vi "main.vi"() -> ()   [LabVIEW 2012]
uses:
  <vilib>/addons/_office/_wordsub.llb/font.ctl
  <vilib>/Utility/miscctls.llb/LVRowAndColumnTypeDef.ctl
  <vilib>/Instr/_visa.llb/VISA Configure Serial Port (Instr).vi
  <vilib>/vision/NI_Vision_Development_Module.lvlib
panel:
  in  "Algorithm":enum32{"Block Matching Algorithm"}(tab)
  in  "Correspondence Options BM":T1={"Method"=0, "Window Size"=25.0, "Minimum Disparity"=0.0, "Number of Disparity"=192.0, "Left - Right Check"=5.0, "Subpixel"=TRUE, "Invalid Disparity Replace Value"=-16.0} caption="Correspondence Options" {"Method" items=["SAD"]; "Number of Disparity" min=16.0 step=16.0; "Window Size" min=5.0 max=255.0 step=2.0}
  in  "Postfilter Options BM":T2={"Texture Threshold"=0.0, "Uniqueness Ratio"=0.0, "Speckle Window Size"=5.0, "Speckle Range"=200.0} caption="Postfilter Options" {"Speckle Range" min=0.0; "Speckle Window Size" min=0.0; "Uniqueness Ratio" min=0.0 max=100.0; "Texture Threshold" min=0.0}
  in  "Prefilter Options":T3={"Filter Type"=2, "Filter Size"=11.0, "Filter Cap"=31.0} {"Filter Type" items=["None", "Normal Response", "Sobel"]; "Filter Cap" min=1.0 max=63.0; "Filter Size" min=5.0 max=255.0 step=2.0}
  in  "Display":enum16{"Disparity Image", "Depth Image"}(ring)=enum."Depth Image"
  in  "示例图片":i32(slide) min=0 max=4 step=1 scale=0.0..4.0
  in  "开关":bool
  in  "Exit":bool
  in  "Interpolate Disparity":bool=TRUE
  in  "Depth Control":cluster{"Min Depth":dbl, "Max Depth":dbl}={"Min Depth"=0.0, "Max Depth"=40.0} {"Max Depth" min=-1.0; "Min Depth" min=-1.0}
  in  "报表信息":cluster{"font":T4, "字符串":string}={"font"={"font name"="", "font size"=12.0, "bold"=2, "italic"=2, "underline"=2, "strike through"=2, "font color"=16777222}, "字符串"=""} {"font"."font size" format="%0.2f"; "font"."strike through" items=["Strk Unchanged", "Strk Yes", "Strk No"]; "font"."underline" items=["Und Unchanged", "Und Yes", "Und No"]; "font"."italic" items=["Ital Unchanged", "Ital Yes", "Ital No"]; "font"."bold" items=["Bold Unchanged", "Bold Yes", "Bold No"]}
  in  "表格":T5={"auto format"=11, "font"={"font name"="", "font size"=0.0, "bold"=0, "italic"=0, "underline"=0, "strike through"=0, "font color"=0}, "表格 2"=[["", "", "", "", "", ""], ["2", "2.5", "7.6", "6.5", "", ""], ["", "", "", "", "", ""], ["", "", "", "", "", ""], ["", "", "", "", "", ""], ["", "", "", "", "", ""]]} {"auto format" items=["xlRangeAutoFormat3DEffects1"=13, "xlRangeAutoFormat3DEffects2"=14, "xlRangeAutoFormatAccounting1"=4, "xlRangeAutoFormatAccounting2"=5, "xlRangeAutoFormatAccounting3"=6, "xlRangeAutoFormatAccounting4"=17, "xlRangeAutoFormatClassic1"=1, "xlRangeAutoFormatClassic2"=2, "xlRangeAutoFormatClassic3"=3, "xlRangeAutoFormatColor1"=7, "xlRangeAutoFormatColor2"=8, "xlRangeAutoFormatColor3"=9, "xlRangeAutoFormatList1"=10, "xlRangeAutoFormatList2"=11, "xlRangeAutoFormatList3"=12, "xlRangeAutoFormatLocalFormat1"=15, "xlRangeAutoFormatLocalFormat2"=16, "xlRangeAutoFormatLocalFormat3"=19, "xlRangeAutoFormatLocalFormat4"=20, "xlRangeAutoFormatReport1"=21, "xlRangeAutoFormatReport2"=22, "xlRangeAutoFormatReport3"=23, "xlRangeAutoFormatReport4"=24, "xlRangeAutoFormatReport5"=25, "xlRangeAutoFormatReport6"=26, "xlRangeAutoFormatReport7"=27, "xlRangeAutoFormatReport8"=28, "xlRangeAutoFormatReport9"=29, "xlRangeAutoFormatReport10"=30, "xlRangeAutoFormatClassicPivotTable"=31, "xlRangeAutoFormatTable1"=32, "xlRangeAutoFormatTable2"=33, "xlRangeAutoFormatTable3"=34, "xlRangeAutoFormatTable4"=35, "xlRangeAutoFormatTable5"=36, "xlRangeAutoFormatTable6"=37, "xlRangeAutoFormatTable7"=38, "xlRangeAutoFormatTable8"=39, "xlRangeAutoFormatTable9"=40, "xlRangeAutoFormatTable10"=41, "xlRangeAutoFormatPTNone"=42, "xlRangeAutoFormatNone"=-4142, "xlRangeAutoFormatSimple"=-4154]; "font"."font size" format="%0.2f"; "font"."strike through" items=["Strk Unchanged", "Strk Yes", "Strk No"]; "font"."underline" items=["Und Unchanged", "Und Yes", "Und No"]; "font"."italic" items=["Ital Unchanged", "Ital Yes", "Ital No"]; "font"."bold" items=["Bold Unchanged", "Bold Yes", "Bold No"]}
  in  "内部数据显示栏值":string[][](array[string])
  out "内部数据数组":string[](array[string])
  out "Y轴（时间）":dbl
  in  "数组":dbl[][](array[numeric])=[[0.0], [0.0], [0.0], [0.0]]
  out "环境数据数组":string[](array[string])
  in  "环境数据显示栏值":string[][](array[string])
  out "Calibrating":bool=TRUE
  in  "Clean":bool
  out "报警计数":dbl
  out "果实报警数组":string[](array[string])
  out "问题叶片报警数组":string[](array[string])
  in  "颜色簇":T6={"报警没确认"=15663104, "背景色"=16448250, "消除没确认"=16777224, "报警已确认"=15331072}
  in  "消除未确认行号数组":dbl[](array[numeric])
  in  "报警已确认行号数组":dbl[](array[numeric])
  in  "报警没确认行号数组":dbl[](array[numeric])
  in  "数据显示栏值":string[][](array[string])
  in  "stop":bool
  in  "主选项卡":enum32{"主控制面板", "记录", "设置"}(tab)
  in  "子选项卡":enum32{"主监视界面", "环境数据监视界面", "内部数据监视界面", "地图"}(tab)
  in  "行驶控制":T7 {"距离" scale=0.0..50.0; "方向" scale=0.36..360.0}
  in  "测试图片":i8(slide) scale=0.0..5.0
  in  "主摄像头开关":bool
  out "花蕾":bool
  out "花朵":bool
  out "问题叶片":bool
  out "正常叶片":bool
  out "未成熟果实":bool
  out "果实":bool
  out "花蕾":dbl
  out "花朵":dbl
  out "问题叶片":dbl
  out "正常叶片":dbl
  out "未成熟果实":dbl
  out "果实":dbl
  out "主摄像头":T8(plugin-control)
  out "通信状态":T9
  out "GPS":T10={"状态"="无效GPS", "经度"="117.124598", "纬度"="34.176800", "UTC"="08时02分46秒"}
  in  "运行状态":T11={"开始时间"="00:00", "停止时间"="00:00", "小车状态"=FALSE}
  out "环境数据":T12
  out "内部数据":cluster{"电量":T13} {"电量" scale=0.0..100.0}
  in  "当前报警":i32(listbox)
  out "环境数据":dbl[][](graph)
  in  "环境数据":i32(listbox)
  in  "内部数据":i32(listbox)
  in  "WebBrowser":refnum<k7>(container) caption="地图显示窗口"
  in  "报警显示选项卡":enum32{"报警", "数据"}(tab)
  in  "当前报警列表框":i32(listbox)
  out "Rar":bool
  out "Pics":bool
  out "Execel":bool
  out "Html":bool
  in  "上传至服务器":bool
  in  "写入数据库":bool
  in  "生成报表":bool
  in  "设置选项卡":T14(tab)
  out "报警设置":i32(listbox)
  out "actual data":string
  in  "GPS状态":string[](array[string])=["初始化", "单点定位", "差分定位", "无效GPS", "固定解", "浮点解", "正在估算"]
  out "状态":string
  out "UTC时间":string
  out "GPGGA":string
  out "经度":string
  out "纬度":string
  in  "VISA resource name":refnum<visa-resource-name>="COM5"
  in  "baud rate (9600)":u32=9600
  in  "确定按钮":bool
  in  "从机数据地址":string="00"
  out "Modbus报文":string
  out "值":dbl
  in  "VISA resource name for Modbus":refnum<visa-resource-name>="COM5"
  out "发生报警":bool
  in  "报警上限":dbl(slide)=81.63265306122449 scale=0.0..100.0
  out "温度计":dbl(slide)=52.47484062973238 scale=0.0..80.0
  in  "stop 2":bool
  in  "清除报警":bool
  out "报警历史":string[][](table)
  out "报警数":i32
  out "湿度计":dbl(slide)=52.47484062973238 scale=0.0..100.0
  out "气压计":dbl(slide)=52.47484062973238 scale=0.0..120.0
  out "光度计":dbl(slide)=52.47484062973238 scale=0.0..200.0
  out "时间标识":timestamp
  out "时间字符串":string
  out "日期字符串":string
  out "Right Image":T8(plugin-control)
  out "Left Image":T8(plugin-control)
  out "Image":sgl[][](graph) caption="Depth Image"
  out "Depth":dbl caption="inches"
  # "LX"
  # "kPa"
  # "%"
  # "°C"
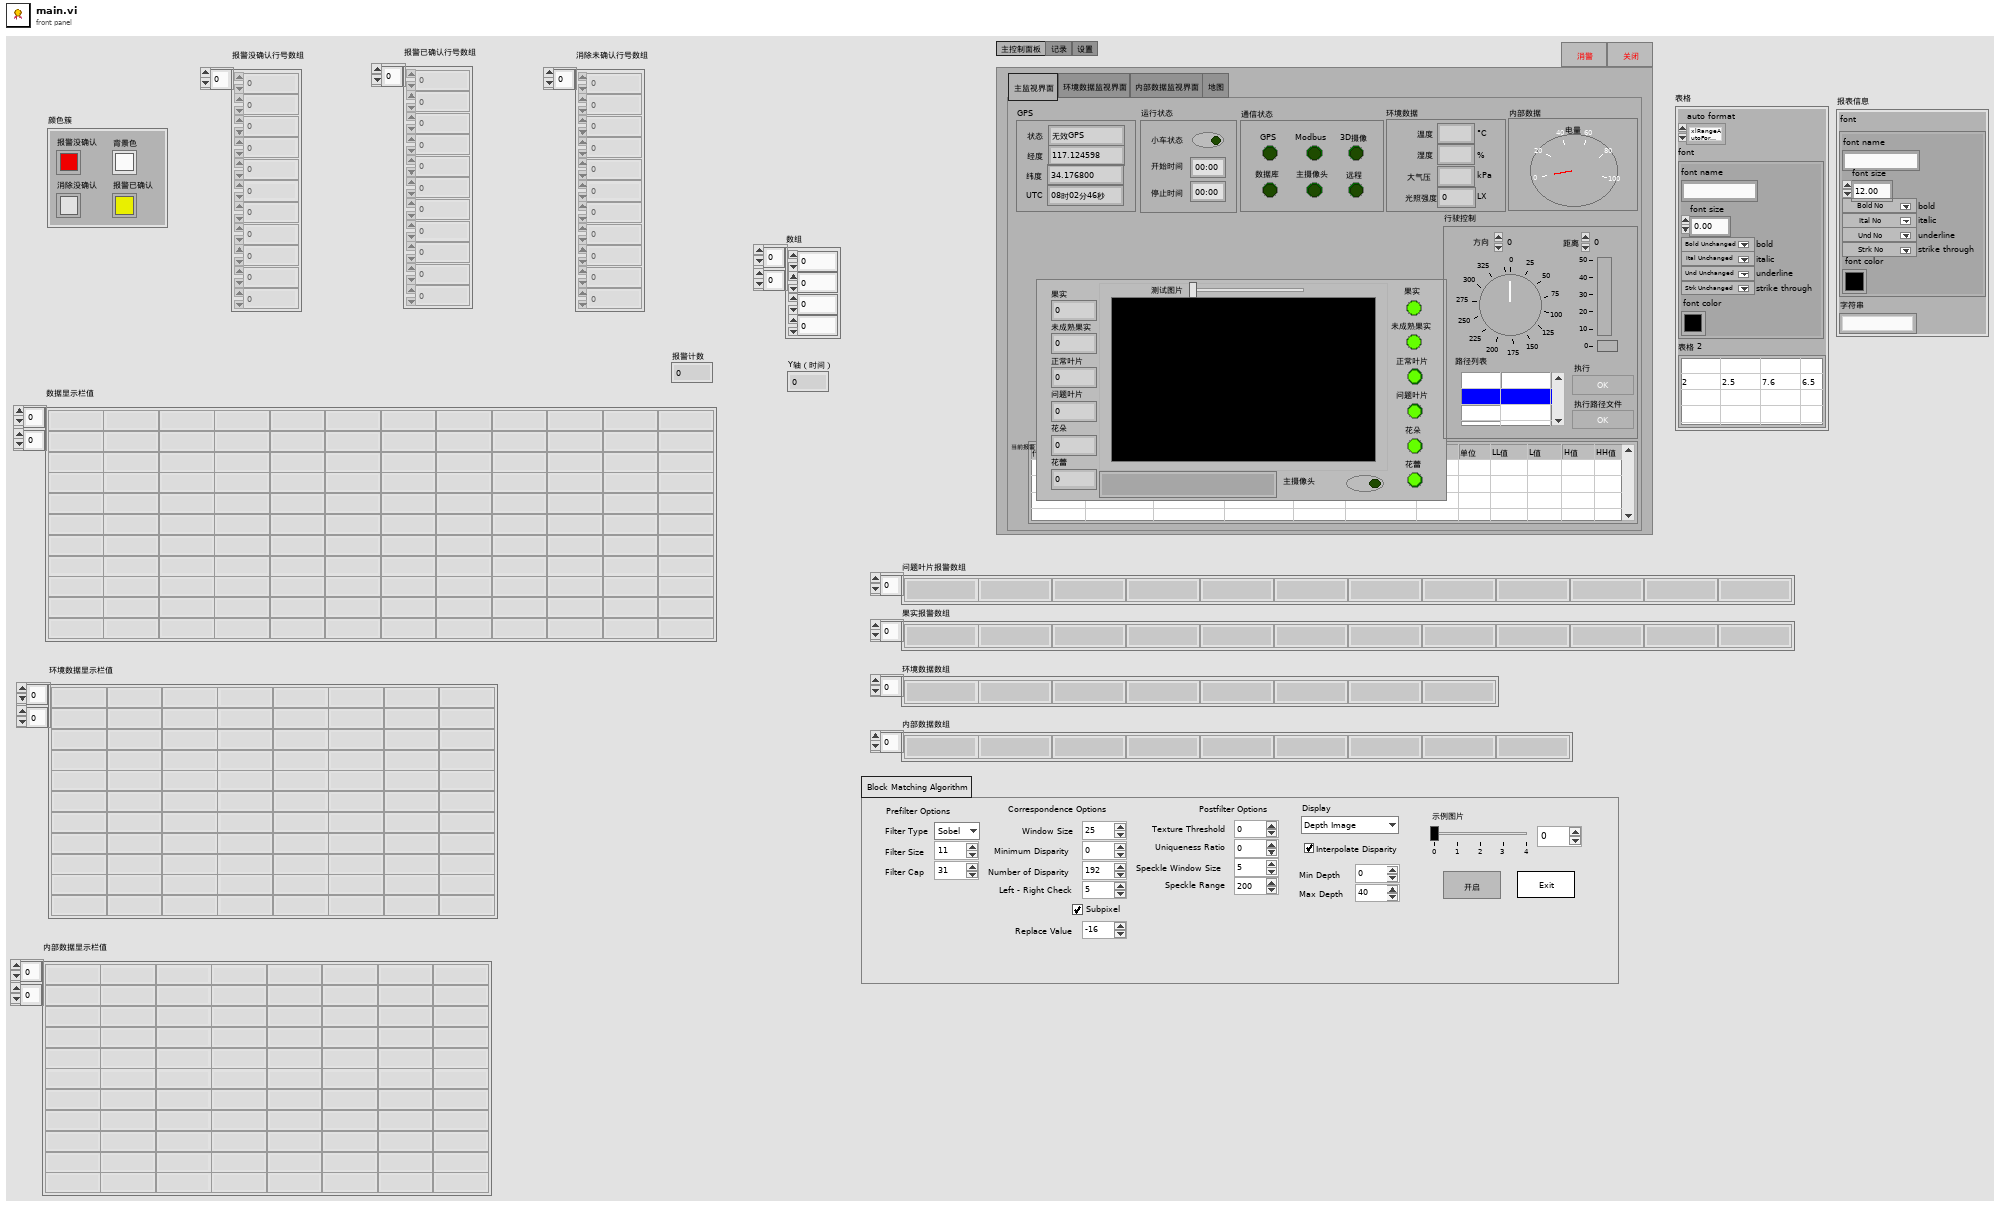
[diagram p1: front panel]
types:
  T1 = cluster{"Method":u16, "Window Size":dbl, "Minimum Disparity":dbl, "Number of Disparity":dbl, "Left - Right Check":dbl, "Subpixel":bool, "Invalid Disparity Replace Value":dbl}
  T2 = cluster{"Texture Threshold":dbl, "Uniqueness Ratio":dbl, "Speckle Window Size":dbl, "Speckle Range":dbl}
  T3 = cluster{"Filter Type":u16, "Filter Size":dbl, "Filter Cap":dbl}
  T4 = typedef "font.ctl" = cluster{"font name":string, "font size":dbl, "bold":u16, "italic":u16, "underline":u16, "strike through":u16, "font color":u32}
  T5 = cluster{"auto format":i32, "font":T4, "表格 2":string[][]}
  T6 = cluster{"报警没确认":u32, "背景色":u32, "消除没确认":u32, "报警已确认":u32}
  T7 = cluster{"方向":i32, "距离":i32, "路径列表":i32, "执行":bool, "执行路径文件":bool}
  T8 = typedef "IMAQ Image.ctl" = refnum<image>
  T9 = cluster{"GPS":bool, "数据库":bool, "Modbus":bool, "主摄像头":bool, "3D摄像":bool, "远程":bool}
  T10 = cluster{"状态":string, "经度":string, "纬度":string, "UTC":string}
  T11 = cluster{"开始时间":string, "停止时间":string, "小车状态":bool}
  T12 = cluster{"温度":dbl, "湿度":dbl, "大气压":dbl, "光照强度":dbl}
  T13 = typedef "电量.ctl" = dbl
  T14 = enum32{"报警值状态", "GPS状态", "Modbus状态", "时间状态", "3D摄像"}
  T15 = typedef "Calibration Reference Points.ctl" = cluster{"Pixel Coordinates":cluster{"X":dbl, "Y":dbl}[], "Real World Coordinates":cluster{"X":dbl, "Y":dbl}[], "Unit":T16, "Image Size":cluster{"X":u32, "Y":u32}}
  T16 = typedef "Image Unit" = enum32{"Undefined", "Angström", "Micrometer", "Millimeter", "Centimeter", "Meter", "Kilometer", "Microinch", "Inch", "Feet", "Nautical miles", "Standard miles", "Steps"}
  T17 = typedef "IMAQ Binocular Stereo Session.ctl" = refnum<k1>
  T18 = typedef "Image Type" = u32
  T19 = typedef "LVPoint32TypeDef.ctl" = cluster{"Horizontal":i32, "Vertical":i32}
  T20 = cluster{"Number of Disparity":dbl, "Number of Disparity":dbl}
  T21 = typedef "LVRowAndColumnTypeDef.ctl" = cluster{"Row":i32, "Column":i32}
  T22 = cluster{"状态":string, "经度":string, "纬度":string, "UTC时间":string}
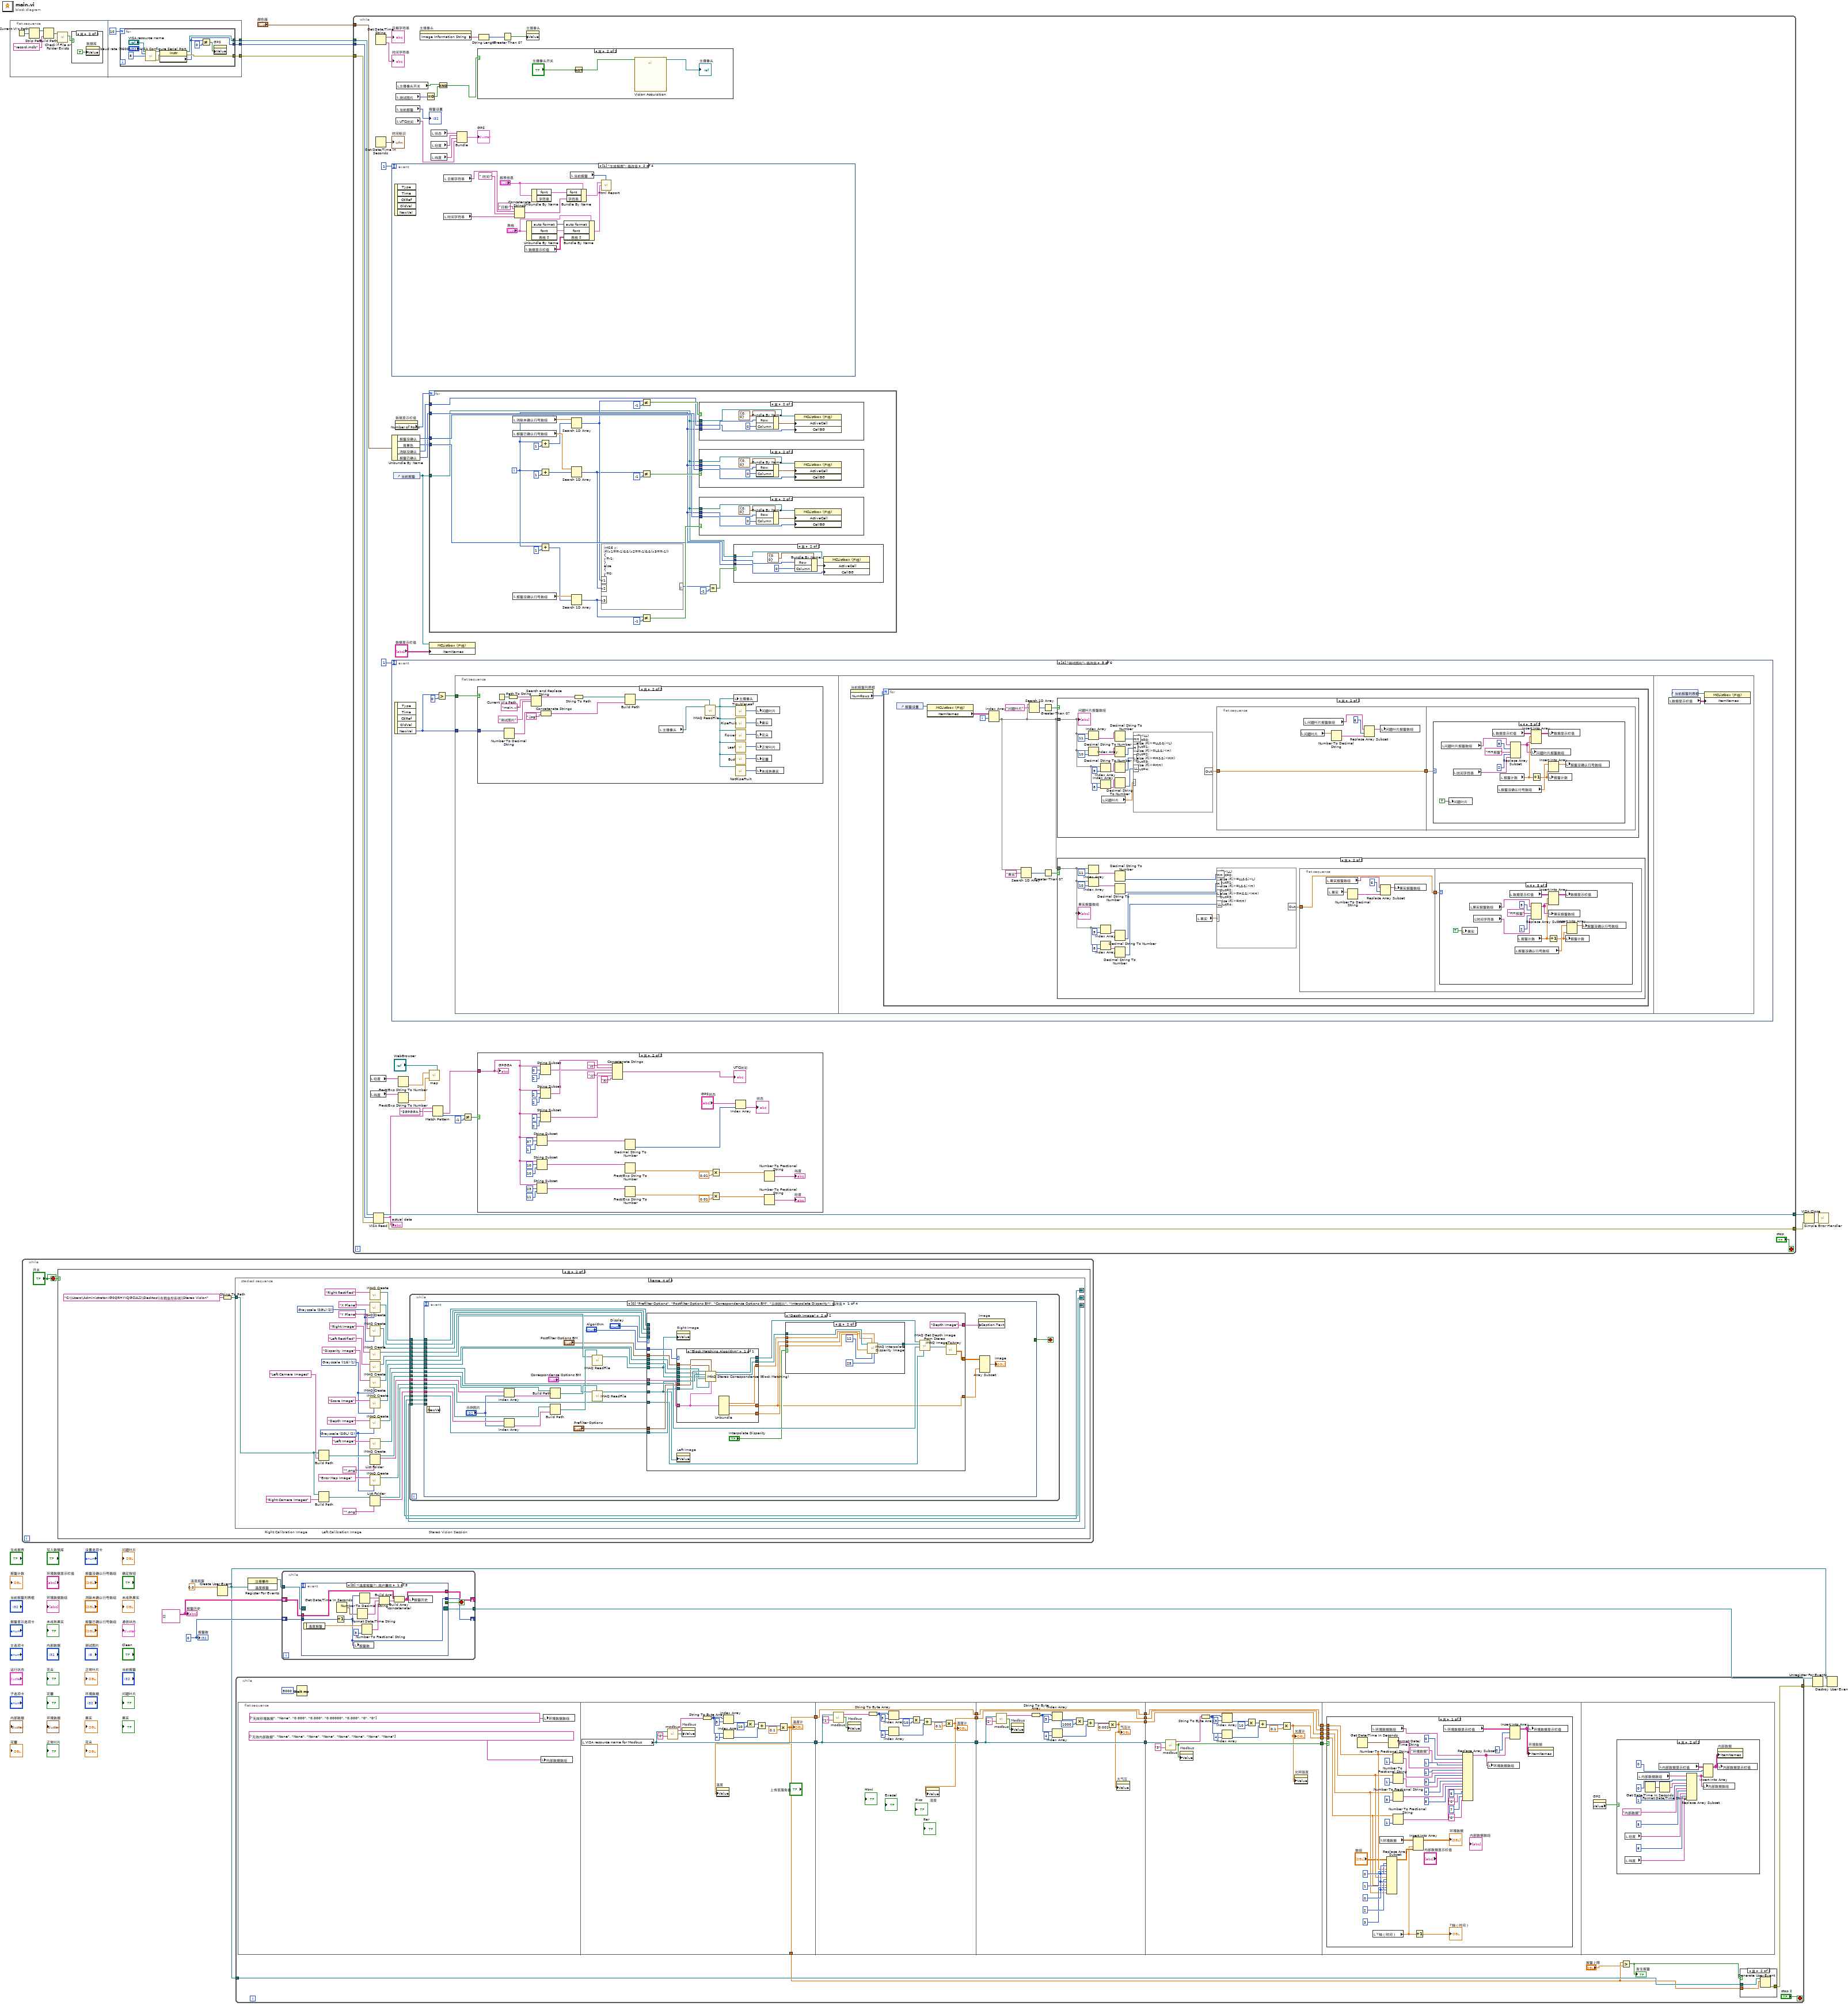
[diagram p0: block diagram]
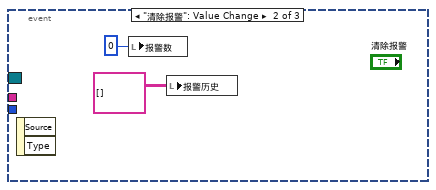
[diagram p2: hidden frame]
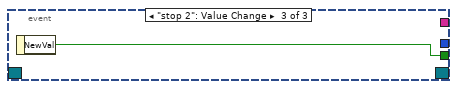
[diagram p3: hidden frame]
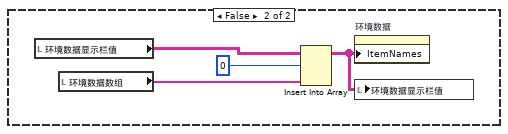
[diagram p4: hidden frame]
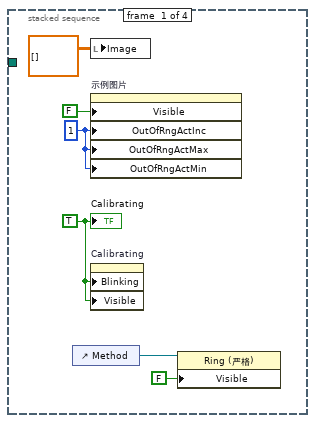
[diagram p8: hidden frame]
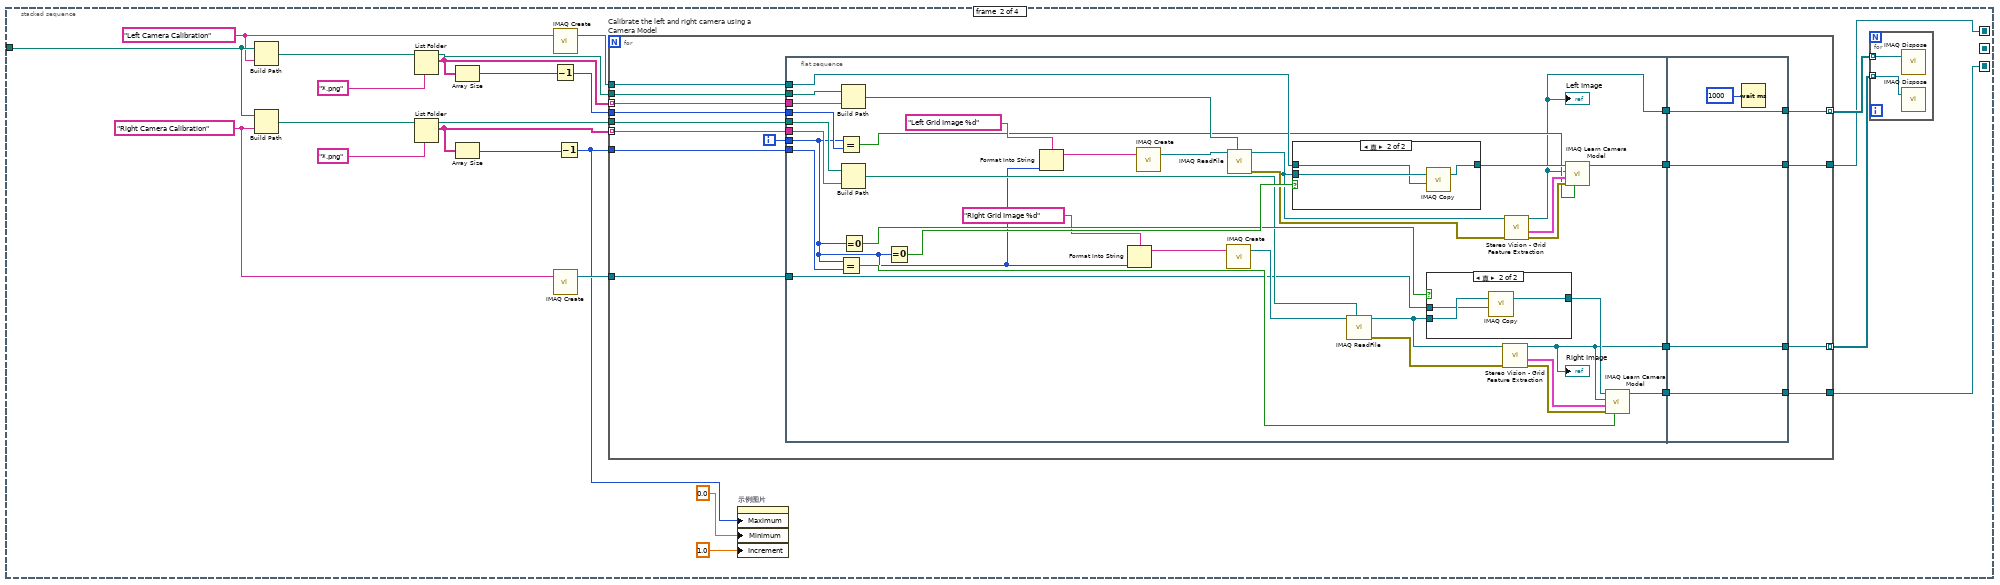
[diagram p9: hidden frame]
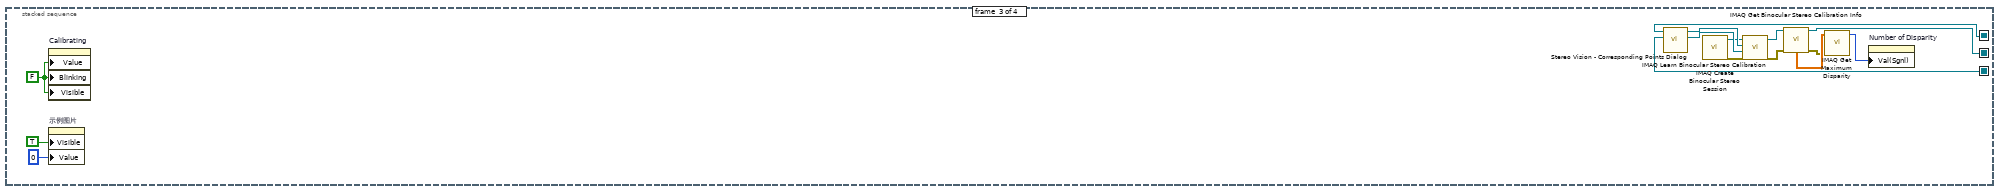
[diagram p12: hidden frame]
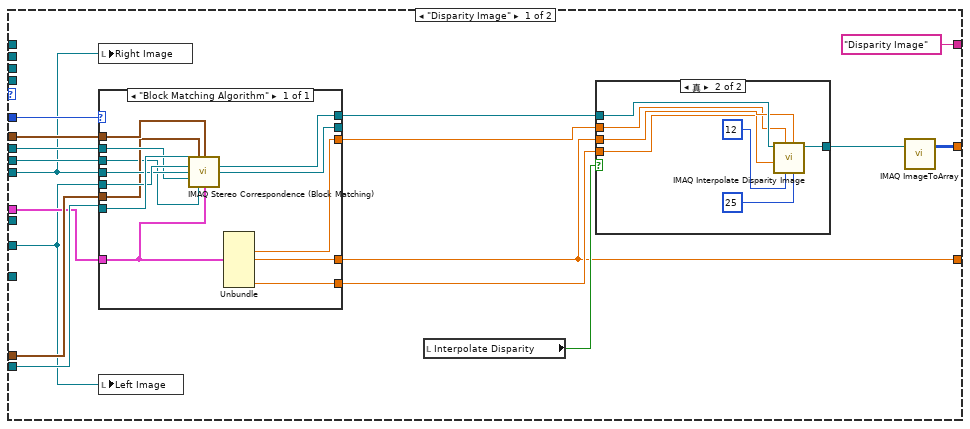
[diagram p13: hidden frame]
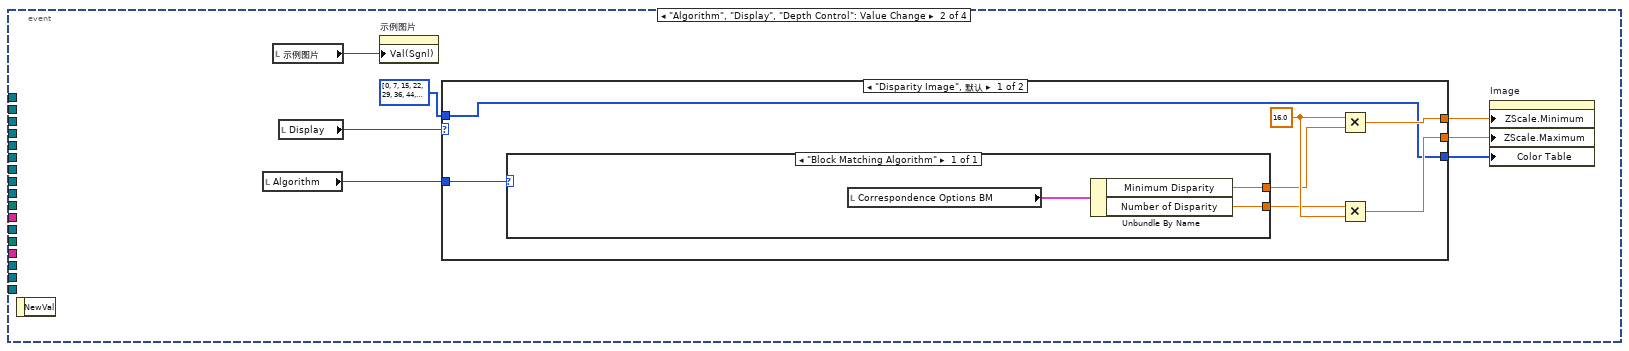
[diagram p16: hidden frame]
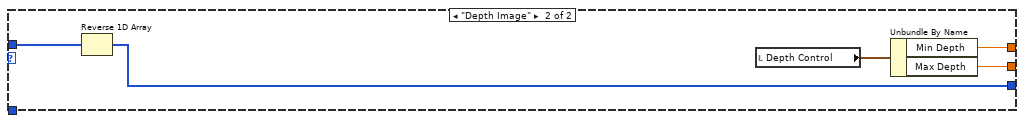
[diagram p17: hidden frame]
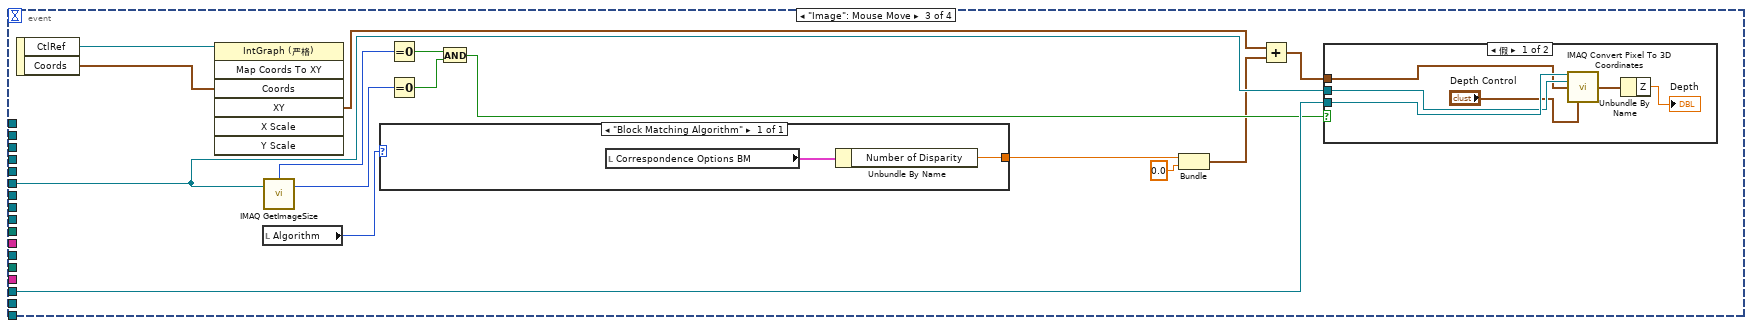
[diagram p18: hidden frame]
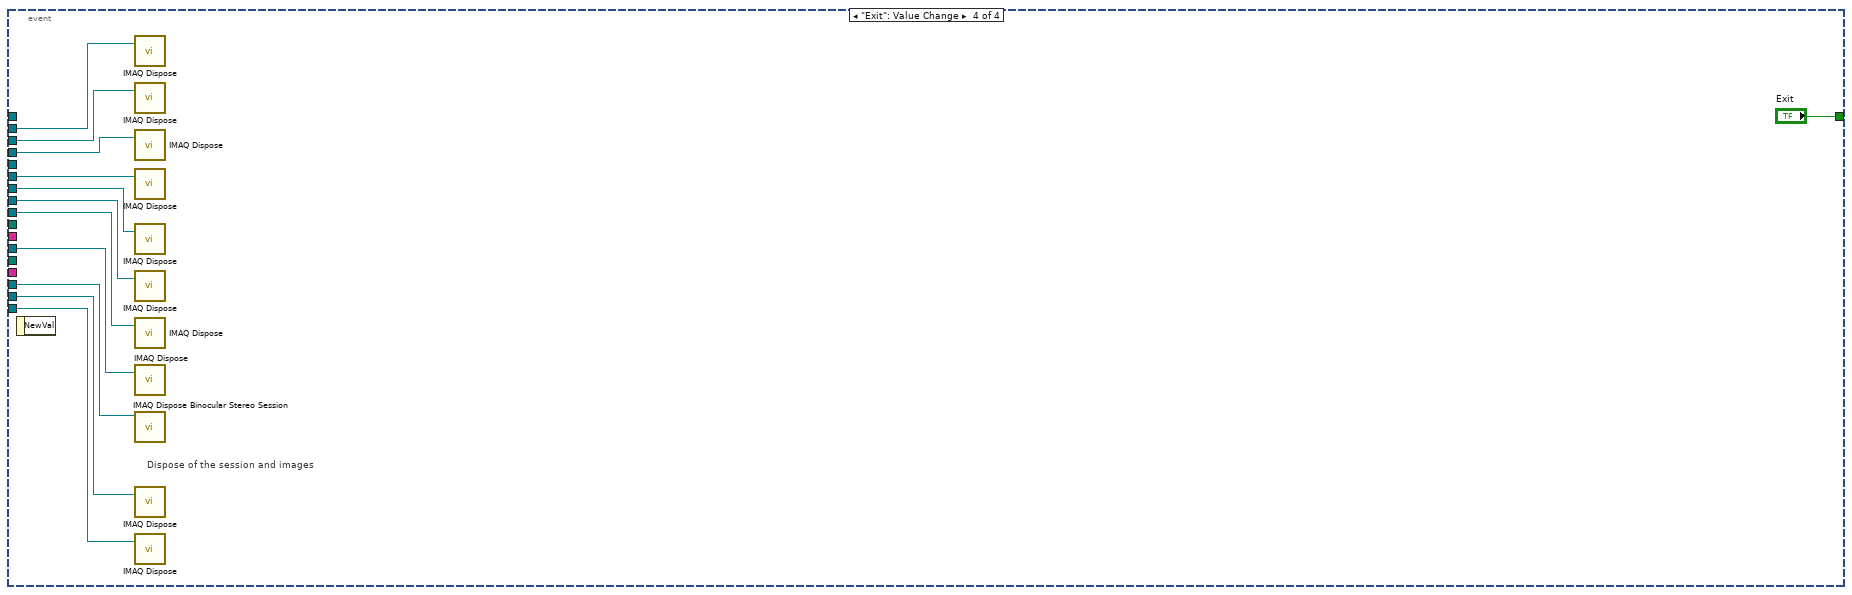
[diagram p20: hidden frame]
diagram:
  w6 = string[][] [] ("报警历史")
  w8 = 0.0  # 温度报警
  w4 = 0
  n1 = flat-sequence {
    tunnel: [w26] -> w12
    tunnel: [w25] -> w11
    tunnel: [w24] -> w10
    frame #0 {
      n2 = Current VI's Path() -> (path=w18:path)
      n3 = Strip Path(path=w18) -> (stripped path=w19:path)  [unwired: 1 out]
      n4 = Build Path(base path=w19, name or relative path="record.mdb") -> (appended path=w20:path)
      n5 = call <vilib>:"Check if File or Folder Exists.vi"("path"=w20) -> ("file or folder exists?"=w16:bool)  [unwired: 8 in, 2 out]
      n6 = case shown="真" w16 {
        frame False {
          n7 = property on="数据库" class="Bool (严格)"("Value"=FALSE) -> ()  [unwired: 2 in, 2 out]
        }
        frame True {
          n8 = property on="数据库" class="Bool (严格)"("Value"=TRUE) -> ()  [unwired: 2 in, 2 out]
        }
      }
    }
    frame #1 {
      n9 = for {
        N: 10 ("offset (0)") -> [_]
        tunnel: [w32] -> w26
        tunnel: [w30] -> w24
        tunnel: [w31] -> w25
        n10 = call-poly "VISA Configure Serial Port"("VISA resource name"="VISA resource name", "baud rate (9600)"="baud rate (9600)", "data bits (8)"=u16 8) -> ("VISA resource name out"=w28:refnum<visa-resource-name>, "error out"=w36:errorcluster)  [unwired: 3 in, 8 out]
        n11 = property class="Instr"(reference=w28, error in=w36) -> (reference out=w32:refnum<visa-resource-name>, error out=w31:errorcluster, "Serial Settings:Number of Bytes at Serial Port"=w30:u32)
        n12 = Not Equal?(x=w30, y=u32 0) -> (x != y?=w27:bool)
        n13 = property on="GPS" class="Bool (严格)"("Value"=w27) -> ()  [unwired: 2 in, 2 out]
      }
    }
  }
  n14 = while {
    stop <- "开关" stop-if-true
    n15 = case shown="真" "开关" {
      frame False {
      }
      frame True {
        # "Stereo Vision Session"
        # "Right Calibration Image"
        # "Left Calibration Image"
        n16 = String To Path(string="C:\\Users\\Administrator.IG0QRHYICJGCULZ\\Desktop\\车载监控系统\\Stereo Vision" ("name or relative path")) -> (path=w38:path)
        n17 = stacked-sequence {
          seq-local: [_ w53 _ _] -> [_ _ w139 w155]
          seq-local: [_ w52 _ _] -> [_ _ w138 w154]
          seq-local: [_ _ w137 _] -> [_ _ _ w153]
          tunnel: w38 -> [_ w65 _ w187]
          frame #0 {
            w43 = u8 1 ("Response to Value Outside Limits:Maximum")
            w44 = TRUE ("Calibrating")
            n18 = control-ref of="Method"() -> (w42:refnum<vi>)
            n19 = local write "Image"(sgl[][] [] ("Image")) -> ()
            n20 = property on="示例图片" class="Slide (严格)"("Visible"=FALSE, "OutOfRngActInc"=w43, "OutOfRngActMax"=w43, "OutOfRngActMin"=w43) -> ()  [unwired: 2 in, 2 out]
            n21 = property on="Calibrating" class="Bool (严格)"("Blinking"=w44, "Visible"=w44) -> ()  [unwired: 2 in, 2 out]
            n22 = property class="Ring (严格)"(reference=w42, "Visible"=FALSE) -> ()  [unwired: 1 in, 2 out]
            "Calibrating" <- w44
          }
          frame #1 {
            w63 = "Right Camera Calibration" ("name or relative path")
            w64 = "Left Camera Calibration" ("name or relative path")
            n23 = Build Path(base path=w65, name or relative path=w64) -> (appended path=w68:path)
            n24 = Build Path(base path=w65, name or relative path=w63) -> (appended path=w66:path)
            n25 = List Folder(path=w68, pattern="*.png") -> (path out=w62:path, filenames=w59:string[])  [unwired: 1 in, 3 out]
            n26 = List Folder(path=w66, pattern="*.png") -> (path out=w61:path, filenames=w56:string[])  [unwired: 1 in, 3 out]
            n27 = Array Size(array=w59) -> (size(s)=w67:i32)
            n28 = Array Size(array=w56) -> (size(s)=w51:i32)
            n29 = call "IMAQ Create"("Image Name"=w64) -> ("New Image"=w60:T8)  [unwired: 3 in, 2 out]
            n30 = Decrement(x=w67) -> (x-1=w58:i32)
            n31 = call "IMAQ Create"("Image Name"=w63) -> ("New Image"=w57:T8)  [unwired: 3 in, 2 out]
            n32 = Decrement(x=w51) -> (x-1=w50:i32)
            n33 = for "Calibrate the left and right camera using a Camera Model" {
              tunnel: w59 -> [w86] mode=indexing
              tunnel: w56 -> [w81] mode=indexing
              tunnel: w62 -> [w87]
              tunnel: w61 -> [w82]
              tunnel: w60 -> [w85]
              tunnel: [w84] -> w53
              tunnel: w58 -> [w83]
              tunnel: [w80] -> w52
              tunnel: w57 -> [w79]
              tunnel: w50 -> [w78]
              tunnel: [w77] -> w54 mode=indexing
              tunnel: [w76] -> w55 mode=indexing
              i -> [w75]
              n34 = flat-sequence {
                tunnel: w87 -> [w118]
                tunnel: w86 -> [w116]
                tunnel: w85 -> [w114]
                tunnel: w83 -> [w109]
                tunnel: w82 -> [w97]
                tunnel: w81 -> [w96]
                tunnel: w79 -> [w94]
                tunnel: w78 -> [w93]
                tunnel: w75 -> [w92]
                tunnel: [w110] -> w74
                tunnel: [w95] -> w73
                tunnel: [w88] -> w72
                tunnel: [w90] -> w71
                tunnel: [w132] -> w76
                tunnel: [w133] -> w77
                tunnel: [w134] -> w80
                tunnel: [w135] -> w84
                tunnel: w74 -> [w135]
                tunnel: w73 -> [w134]
                tunnel: w72 -> [w133]
                tunnel: w71 -> [w132]
                frame #0 {
                  n35 = Equal?(x=w92, y=w109) -> (x = y?=w108:bool)
                  n36 = Equal?(x=w92, y=w93) -> (x = y?=w107:bool)
                  n37 = Build Path(base path=w118, name or relative path=w116) -> (appended path=w119:path)
                  n38 = Build Path(base path=w97, name or relative path=w96) -> (appended path=w101:path)
                  n39 = Equal To 0?(x=w92) -> (x = 0?=w104:bool)
                  n40 = Equal To 0?(x=w92) -> (x = 0?=w113:bool)
                  n41 = Format Into String(format string="Left Grid Image %d" ("name or relative path"), w92) -> (resulting string=w115:string)  [unwired: 2 in, 1 out]
                  n42 = Format Into String(format string="Right Grid Image %d" ("name or relative path"), w92) -> (resulting string=w103:string)  [unwired: 2 in, 1 out]
                  n43 = call "IMAQ Create"("Image Name"=w115) -> ("New Image"=w122:T8)  [unwired: 3 in, 2 out]
                  n44 = call "IMAQ Create"("Image Name"=w103) -> ("New Image"=w98:T8)  [unwired: 3 in, 2 out]
                  n45 = call "IMAQ ReadFile"("File Path"=w119, "Image"=w122) -> ("error out"=w111:errorcluster, "Image Out"=w91:T8)  [unwired: 3 in, 5 out]
                  n46 = case shown="真" w113 {
                    tunnel: w91 -> [_ w130]
                    tunnel: w114 -> [w127 w129]
                    tunnel: [w127 w128] -> w112
                    frame False {
                    }
                    frame True {
                      n47 = call "IMAQ Copy"("Image Dst"=w129, "Image Src"=w130) -> ("Image Dst Out"=w128:T8)  [unwired: 1 in, 4 out]
                    }
                  }
                  n48 = call "IMAQ ReadFile"("File Path"=w101, "Image"=w98) -> ("error out"=w106:errorcluster, "Image Out"=w89:T8)  [unwired: 3 in, 5 out]
                  n49 = case shown="真" w104 {
                    tunnel: w89 -> [_ w126]
                    tunnel: w94 -> [w123 w125]
                    tunnel: [w123 w124] -> w105
                    frame False {
                    }
                    frame True {
                      n50 = call "IMAQ Copy"("Image Dst"=w125, "Image Src"=w126) -> ("Image Dst Out"=w124:T8)  [unwired: 1 in, 4 out]
                    }
                  }
                  n51 = call "Stereo Vision - Grid Feature Extraction.vi"("error in (no error)"=w106, "Image in"=w89) -> ("error out"=w99:errorcluster, "Reference Points"=w100:T15, "Image (dup)"=w88:T8)  [unwired: 7 out]
                  "Right Image" <- w88
                  n52 = call "Stereo Vision - Grid Feature Extraction.vi"("error in (no error)"=w111, "Image in"=w91) -> ("error out"=w121:errorcluster, "Reference Points"=w120:T15, "Image (dup)"=w90:T8)  [unwired: 7 out]
                  "Left Image" <- w90
                  n53 = call "IMAQ Learn Camera Model"("Add Points and Learn (True)"=w108, "error in (no error)"=w121, "Reference Points"=w120, "Image"=w90, "Calibration Template Image"=w112) -> ("Calibration Template Image Out"=w110:T8)  [unwired: 1 in, 5 out]
                  n54 = call "IMAQ Learn Camera Model"("Add Points and Learn (True)"=w107, "error in (no error)"=w99, "Reference Points"=w100, "Image"=w88, "Calibration Template Image"=w105) -> ("Calibration Template Image Out"=w95:T8)  [unwired: 1 in, 5 out]
                }
                frame #1 {
                  n55 = Wait (ms)(milliseconds to wait=u32 1000 ("millisecond timer value")) -> ()  [unwired: 1 out]
                }
              }
            }
            n56 = property on="示例图片" class="Slide (严格)"("Maximum"=w50, "Minimum"=0.0 ("Data Entry Limits:Minimum"), "Increment"=1.0 ("Data Entry Limits:Increment")) -> ()  [unwired: 2 in, 2 out]
            n57 = for {
              tunnel: w55 -> [w70] mode=indexing
              tunnel: w54 -> [w69] mode=indexing
              n58 = call "IMAQ Dispose"("Image"=w70) -> ()  [unwired: 2 in, 4 out]
              n59 = call "IMAQ Dispose"("Image"=w69) -> ()  [unwired: 2 in, 4 out]
            }
          }
          frame #2 {
            w150 = FALSE ("Calibrating")
            n60 = property on="Calibrating" class="Bool (严格)"("Value"=w150, "Blinking"=w150, "Visible"=w150) -> ()  [unwired: 2 in, 2 out]
            n61 = property on="示例图片" class="Slide (严格)"("Visible"=TRUE, "Value"=0 ("Value (Signaling)")) -> ()  [unwired: 2 in, 2 out]
            n62 = call "Stereo Vision - Corresponding Points Dialog.vi"("Right Image in"=w138, "Left Image in"=w139) -> ("Right Image out"=w143:T8, "Left Image out"=w142:T8)  [unwired: 8 out]
            n63 = call "IMAQ Create Binocular Stereo Session"() -> ("error out"=w141:errorcluster, "Binocular Stereo Session Out"=w140:T17)  [unwired: 1 in, 9 out]
            n64 = call "IMAQ Learn Binocular Stereo Calibration"("error in (no error)"=w141, "Right Calibration Template"=w143, "Left Calibration Template"=w142, "Binocular Stereo Session"=w140) -> ("error out"=w147:errorcluster, "Binocular Stereo Session (dup)"=w146:T17)  [unwired: 1 in, 5 out]
            n65 = call "IMAQ Get Binocular Stereo Calibration Info"("Binocular Stereo Session"=w146, "error in (no error)"=w147) -> ("Binocular Stereo Session (dup)"=w137:T17, "Q Matrix"=w145:dbl[][], "error out"=w144:errorcluster)  [unwired: 11 out]
            n66 = call "IMAQ Get Maximum Disparity"("error in (no error)"=w144, "Q Matrix"=w145) -> ("Max. Disparity"=w136:i32)  [unwired: 2 in, 7 out]
            n67 = property on="Number of Disparity" class="DigNum (严格)"("Val(Sgnl)"=w136) -> ()  [unwired: 2 in, 2 out]
          }
          frame #3 {
            w160 = T18 2 items=["Grayscale (U8)", "Grayscale (I16)", "Grayscale (SGL)", "Complex (CSG)", "RGB (U32)", "HSL (U32)", "RGB (U64)", "Grayscale (U16)"] ("Image Type")
            w161 = T18 2 items=["Grayscale (U8)", "Grayscale (I16)", "Grayscale (SGL)", "Complex (CSG)", "RGB (U32)", "HSL (U32)", "RGB (U64)", "Grayscale (U16)"] ("Image Type")
            w162 = T18 1 items=["Grayscale (U8)", "Grayscale (I16)", "Grayscale (SGL)", "Complex (CSG)", "RGB (U32)", "HSL (U32)", "RGB (U64)", "Grayscale (U16)"] ("Image Type")
            n68 = Build Path(base path=w187, name or relative path="Left Camera Images") -> (appended path=w186:path)
            n69 = Build Path(base path=w187, name or relative path="Right Camera Images") -> (appended path=w183:path)
            n70 = call "IMAQ Create"("Image Name"="Right Rectified") -> ("New Image"=w156:T8)  [unwired: 3 in, 2 out]
            n71 = call "IMAQ Create"("Image Name"="X Plane", "Image Type"=w160) -> ("New Image"=w164:T8)  [unwired: 2 in, 2 out]
            n72 = call "IMAQ Create"("Image Name"="Y Plane", "Image Type"=w160) -> ("New Image"=w163:T8)  [unwired: 2 in, 2 out]
            n73 = call "IMAQ Create"("Image Name"="Right Image") -> ("New Image"=w175:T8)  [unwired: 3 in, 2 out]
            n74 = call "IMAQ Create"("Image Name"="Left Rectified") -> ("New Image"=w157:T8)  [unwired: 3 in, 2 out]
            n75 = call "IMAQ Create"("Image Name"="Disparity Image", "Image Type"=w162) -> ("New Image"=w173:T8)  [unwired: 2 in, 2 out]
            n76 = call "IMAQ Create"("Image Name"="Score Image", "Image Type"=w162) -> ("New Image"=w171:T8)  [unwired: 2 in, 2 out]
            n77 = call "IMAQ Create"("Image Name"="Depth Image", "Image Type"=w161) -> ("New Image"=w169:T8)  [unwired: 2 in, 2 out]
            n78 = call "IMAQ Create"("Image Name"="Left Image") -> ("New Image"=w178:T8)  [unwired: 3 in, 2 out]
            n79 = List Folder(path=w186, pattern="*.png") -> (path out=w180:path, filenames=w182:string[])  [unwired: 1 in, 3 out]
            n80 = call "IMAQ Create"("Image Name"="Error Map Image", "Image Type"=w161) -> ("New Image"=w167:T8)  [unwired: 2 in, 2 out]
            n81 = List Folder(path=w183, pattern="*.png") -> (path out=w179:path, filenames=w181:string[])  [unwired: 1 in, 3 out]
            n82 = while {
              tunnel: w182 -> [w205]
              tunnel: w181 -> [w204]
              tunnel: w180 -> [w203]
              tunnel: w179 -> [w202]
              tunnel: w178 -> [w201]
              tunnel: w153 -> [w200]
              tunnel: w175 -> [w199]
              tunnel: w173 -> [w198]
              tunnel: w171 -> [w197]
              tunnel: w169 -> [w196]
              tunnel: w167 -> [w195]
              tunnel: w164 -> [w194]
              tunnel: w163 -> [w193]
              tunnel: w155 -> [w191]
              tunnel: w154 -> [w190]
              tunnel: w157 -> [w189]
              tunnel: w156 -> [w188]
              stop <- w192 stop-if-true
              n83 = event shown="[0] \"Prefilter Options\", \"Postfilter Options BM\", \"Correspondence Options BM\", \"示例图片\", \"Interpolate Disparity\": 值改变" {
                selector: _ -> [_ _ _ _]
                dyn-events: _ -> [_ _ _ _]
                timeout: _ -> [_ _ _ _]
                tunnel: w205 -> [w232 _ _ _]
                tunnel: w204 -> [w230 _ _ _]
                tunnel: w203 -> [w233 _ _ _]
                tunnel: w202 -> [w231 _ _ _]
                tunnel: w201 -> [w228 _ _ w372]
                tunnel: w200 -> [w225 _ w353 w364]
                tunnel: w199 -> [w223 _ _ w371]
                tunnel: w198 -> [w222 _ w352 w370]
                tunnel: w197 -> [w218 _ _ w369]
                tunnel: w196 -> [w217 _ _ w368]
                tunnel: w195 -> [w215 _ _ w367]
                tunnel: w194 -> [w214 _ _ w366]
                tunnel: w193 -> [w213 _ _ w365]
                tunnel: [_ _ _ "Exit"] -> w192
                tunnel: w191 -> [_ _ _ w363]
                tunnel: w190 -> [_ _ _ w362]
                tunnel: w189 -> [w212 _ _ _]
                tunnel: w188 -> [w211 _ _ _]
                event "Prefilter Options", "Postfilter Options BM", "Correspondence Options BM", "示例图片", "Interpolate Disparity": Value Change {
                  n84 = event-data() -> ()  [unwired: 2 out]
                  n85 = Index Array(array=w232, index="示例图片") -> (element=w236:string)
                  n86 = Index Array(array=w230, index="示例图片") -> (element=w235:string)
                  n87 = Build Path(base path=w233, name or relative path=w236) -> (appended path=w234:path)
                  n88 = Build Path(base path=w231, name or relative path=w235) -> (appended path=w224:path)
                  n89 = call "IMAQ ReadFile"("File Path"=w224, "Image"=w223) -> ("Image Out"=w209:T8)  [unwired: 3 in, 6 out]
                  n90 = call "IMAQ ReadFile"("File Path"=w234, "Image"=w228) -> ("Image Out"=w210:T8)  [unwired: 3 in, 6 out]
                  n91 = case shown="\"Depth Image\"" "Display" {
                    tunnel: w225 -> [w251 w290]
                    tunnel: w210 -> [w239 w284]
                    tunnel: w209 -> [w238 w283]
                    tunnel: w222 -> [w250 w289]
                    tunnel: "Algorithm" -> [w247 w293]
                    tunnel: "Postfilter Options BM" -> [w253 w292]
                    tunnel: "Prefilter Options" -> [w252 w291]
                    tunnel: "Correspondence Options BM" -> [w249 w287]
                    tunnel: [w240 w276] -> w208
                    tunnel: ["Disparity Image" ("Caption.Text") "Depth Image" ("Caption.Text")] -> w216
                    tunnel: w218 -> [w246 w288]
                    tunnel: w217 -> [_ w294]
                    tunnel: w215 -> [_ w285]
                    tunnel: w214 -> [_ _]
                    tunnel: w213 -> [_ _]
                    tunnel: w212 -> [_ _]
                    tunnel: w211 -> [_ _]
                    tunnel: [w237 w275] -> w206
                    frame "Disparity Image" {
                      n92 = local write "Right Image"(w238) -> ()
                      n93 = case shown="\"Block Matching Algorithm\"" w247 {
                        tunnel: w251 -> [w274]
                        tunnel: w239 -> [w273]
                        tunnel: w238 -> [w272]
                        tunnel: w250 -> [w271]
                        tunnel: [w270] -> w245
                        tunnel: w253 -> [w269]
                        tunnel: w252 -> [w268]
                        tunnel: w249 -> [w265]
                        tunnel: w246 -> [w267]
                        tunnel: [w266] -> _
                        tunnel: [w262] -> w244
                        tunnel: [w264] -> w243
                        tunnel: [w263] -> w237
                        frame "Block Matching Algorithm" {
                          n94 = call "IMAQ Stereo Correspondence (Block Matching)"("Binocular Stereo Session"=w274, "Prefilter Options"=w268, "Postfilter Options"=w269, "Left Image In"=w273, "Right Image In"=w272, "Disparity Image In"=w271, "Score Image In"=w267, "Correspondence Options"=w265) -> ("Disparity Image Out"=w270:T8, "Score Image Out"=w266:T8)  [unwired: 1 in, 5 out]
                          n95 = Unbundle(w265) -> ("Minimum Disparity"=w264:dbl, "Number of Disparity"=w263:dbl, "Invalid Disparity Replace Value"=w262:dbl)  [unwired: 4 out]
                        }
                      }
                      n96 = local write "Left Image"(w239) -> ()
                      n97 = local read "Interpolate Disparity"() -> (w242:bool)
                      n98 = case shown="真" w242 {
                        tunnel: w245 -> [w254 w261]
                        tunnel: [w254 w260] -> w241
                        tunnel: w237 -> [_ w259]
                        tunnel: w243 -> [_ w258]
                        tunnel: w244 -> [_ w257]
                        frame False {
                        }
                        frame True {
                          n99 = call "IMAQ Interpolate Disparity Image"("Sampling Frequency"=25, "Number of Disparities"=w259, "Order"=12, "Minimum Disparity"=w258, "Invalid Disparity Value"=w257, "Image Src"=w261) -> ("Image Dst Out"=w260:T8)  [unwired: 2 in, 3 out]
                        }
                      }
                      n100 = call "IMAQ ImageToArray"("Image"=w241) -> ("Image Pixels (I16)"=w240:i16[][])  [unwired: 2 in, 5 out]
                    }
                    frame "Depth Image" {
                      n101 = property on="Right Image" class="ImageControl"("Value"=w283) -> ()  [unwired: 2 in, 2 out]
                      n102 = case shown="\"Block Matching Algorithm\"" w293 {
                        tunnel: w290 -> [w316]
                        tunnel: w284 -> [w315]
                        tunnel: w283 -> [w314]
                        tunnel: w289 -> [w313]
                        tunnel: [w312] -> w281
                        tunnel: w292 -> [w311]
                        tunnel: w291 -> [w310]
                        tunnel: w288 -> [w309]
                        tunnel: w287 -> [w307]
                        tunnel: [w308] -> w286
                        tunnel: [w306] -> w280
                        tunnel: [w305] -> w279
                        tunnel: [w304] -> w275
                        frame "Block Matching Algorithm" {
                          n103 = call "IMAQ Stereo Correspondence (Block Matching)"("Binocular Stereo Session"=w316, "Prefilter Options"=w310, "Postfilter Options"=w311, "Left Image In"=w315, "Right Image In"=w314, "Disparity Image In"=w313, "Score Image In"=w309, "Correspondence Options"=w307) -> ("Binocular Stereo Session (dup)"=w308:T17, "Disparity Image Out"=w312:T8)  [unwired: 1 in, 5 out]
                          n104 = Unbundle(w307) -> ("Minimum Disparity"=w305:dbl, "Number of Disparity"=w304:dbl, "Invalid Disparity Replace Value"=w306:dbl)  [unwired: 4 out]
                        }
                      }
                      n105 = property on="Left Image" class="ImageControl"("Value"=w284) -> ()  [unwired: 2 in, 2 out]
                      n106 = case shown="真" "Interpolate Disparity" {
                        tunnel: [w296 w303] -> w282
                        tunnel: w281 -> [w296 w302]
                        tunnel: w280 -> [_ w301]
                        tunnel: w279 -> [_ w300]
                        tunnel: w275 -> [_ w299]
                        frame False {
                        }
                        frame True {
                          n107 = call "IMAQ Interpolate Disparity Image"("Sampling Frequency"=25, "Number of Disparities"=w299, "Order"=12, "Minimum Disparity"=w300, "Invalid Disparity Value"=w301, "Image Src"=w302) -> ("Image Dst Out"=w303:T8)  [unwired: 2 in, 3 out]
                        }
                      }
                      n108 = call "IMAQ Get Depth Image From Stereo"("Error Map In"=w285, "Depth Image In"=w294, "Disparity Image"=w282, "Binocular Stereo Session"=w286) -> ("Depth Image Out"=w277:T8)  [unwired: 3 in, 4 out]
                      n109 = call "IMAQ ImageToArray"("Image"=w277) -> ("Image Pixels (Float)"=w276:sgl[][])  [unwired: 2 in, 5 out]
                    }
                  }
                  n110 = property on="Image" class="IntGraph (严格)"("Caption.Text"=w216) -> ()  [unwired: 2 in, 2 out]
                  n111 = Array Subset(array=w208, index (col)=w206) -> (→"Image":sgl[][])  [unwired: 3 in]
                }
                event "Correspondence Options BM.Minimum Disparity", "Correspondence Options BM.Number of Disparity", "Algorithm", "Display", "Depth Control": Value Change {
                  n112 = event-data() -> ()  [unwired: 2 out]
                  n113 = local read "Algorithm"() -> (w323:enum32{"Block Matching Algorithm"})
                  n114 = local read "示例图片"() -> (w317:i32)
                  n115 = local read "Display"() -> (w320:enum16{"Disparity Image", "Depth Image"})
                  n116 = property on="示例图片" class="Slide (严格)"("Val(Sgnl)"=w317) -> ()  [unwired: 2 in, 2 out]
                  n117 = case shown="\"Disparity Image\", 默认" w320 {
                    tunnel: w323 -> [w330 _]
                    tunnel: [w326 w335] -> w322
                    tunnel: [w325 w334] -> w321
                    tunnel: u32[] [0, 7, 15, 22, 29, 36, 44, 51, 58, 66, 73, 80, 87, 95, 102, 109, 117, 124, 131, 138, 146, 153, 160, 168, 175, 182, 189, 197, 204, 211, 219, 226, 233, 240, 248, 255, 75263, 76799, 78335, 79871, 81407, 82943, 84479, 86015, 87551, 89087, 90623, 92159, 93695, 95231, 96767, 98303, 99839, 101375, 102911, 104447, 105983, 107519, 109055, 110591, 112127, 113663, 115199, 116735, 118271, 119807, 121343, 122879, 124415, 125951, 127487, 129023, 130559, 131069, 131063, 131057, 131051, 131045, 131039, 131033, 131027, 131021, 131015, 131009, 131003, 130997, 130991, 130985, 130979, 130973, 130967, 130961, 130955, 130949, 130943, 130937, 130931, 130925, 130919, 130913, 130907, 130901, 130895, 130889, 130883, 130877, 130871, 130865, 130859, 130853, 130847, 130841, 130835, 130829, 130823, 130817, 524033, 917249, 1310465, 1703681, 2096897, 2490113, 2883329, 3276545, 3669761, 4062977, 4456193, 4849409, 5242625, 5635841, 6029057, 6422273, 6815489, 7208705, 7601921, 7995137, 8388353, 8781569, 9174785, 9568001, 9961217, 10354433, 10747649, 11140865, 11534081, 11927297, 12320513, 12713729, 13106945, 13500161, 13893377, 14286593, 14679809, 15073025, 15466241, 15859457, 16252673, 16645889, 16776449, 16774913, 16773377, 16771841, 16770305, 16768769, 16767233, 16765697, 16762625, 16761089, 16759553, 16758017, 16756481, 16754945, 16753409, 16751873, 16750337, 16748801, 16747265, 16745729, 16744193, 16742657, 16741121, 16739585, 16738049, 16736513, 16734977, 16733441, 16731905, 16730369, 16728833, 16727297, 16725761, 16724225, 16722689, 16721153, 16719617, 16718081, 16716545, 16715009, 16713473, 16711937, 16711937, 16711943, 16711949, 16711955, 16711961, 16711967, 16711973, 16711979, 16711985, 16711991, 16711997, 16712003, 16712009, 16712015, 16712021, 16712027, 16712033, 16712039, 16712045, 16712051, 16712057, 16712063, 16712069, 16712075, 16712081, 16712087, 16712093, 16712099, 16712105, 16712111, 16712117, 16712123, 16712129, 16712135, 16712141, 16712147, 16712153, 16712159, 16712165, 16712171, 16712177, 16712183, 16712189, 16581119, 16187903, 15794687, 15401471, 15008255, 14615039, 14221823, 13828607, 13435391, 13042175, 12648959, 12255743, 11862527] ("appended array") -> [w324 w338]
                    tunnel: [w324 w337] -> w318
                    frame "Disparity Image", Default {
                      w329 = 16.0 ("y")
                      n118 = case shown="\"Block Matching Algorithm\"" w330 {
                        tunnel: [w331] -> w327
                        tunnel: [w332] -> w328
                        frame "Block Matching Algorithm" {
                          n119 = local read "Correspondence Options BM"() -> (w333:T1)
                          n120 = Unbundle By Name(w333) -> ("Minimum Disparity"=w332:dbl, "Number of Disparity"=w331:dbl)
                        }
                      }
                      n121 = Multiply(x=w329, y=w328) -> (x*y=w326:dbl)
                      n122 = Multiply(x=w327, y=w329) -> (x*y=w325:dbl)
                    }
                    frame "Depth Image" {
                      n123 = Reverse 1D Array(array=w338) -> (reversed array=w337:u32[])
                      n124 = local read "Depth Control"() -> (w336:cluster{"Min Depth":dbl, "Max Depth":dbl})
                      n125 = Unbundle By Name(w336) -> ("Min Depth"=w335:dbl, "Max Depth"=w334:dbl)
                    }
                  }
                  n126 = property on="Image" class="IntGraph (严格)"("ZScale.Minimum"=w322, "ZScale.Maximum"=w321, "Color Table"=w318) -> ()  [unwired: 2 in, 2 out]
                }
                event "Image": Mouse Move {
                  n127 = event-data() -> ("CtlRef"=w346:refnum<vi>, "Coords"=w345:T19)  [unwired: 1 out]
                  n128 = invoke class="IntGraph (严格)" method="Map Coords To XY"(reference=w346, "Coords"=w345) -> ("XY"=w341:cluster{"X":dbl, "Y":dbl})  [unwired: 5 in, 6 out]
                  n129 = local read "Algorithm"() -> (w344:enum32{"Block Matching Algorithm"})
                  n130 = call "IMAQ GetImageSize"("Image"=w352) -> ("Y Resolution"=w350:i32, "X Resolution"=w351:i32)  [unwired: 1 in, 3 out]
                  n131 = case shown="\"Block Matching Algorithm\"" w344 {
                    tunnel: [w354] -> w343
                    frame "Block Matching Algorithm" {
                      n132 = local read "Correspondence Options BM"() -> (w355:T1)
                      n133 = Unbundle By Name(w355) -> ("Number of Disparity"=w354:dbl)
                    }
                  }
                  n134 = Equal To 0?(x=w351) -> (x = 0?=w349:bool)
                  n135 = Equal To 0?(x=w350) -> (x = 0?=w348:bool)
                  n136 = And(x=w349, y=w348) -> (x .and. y?=w347:bool)
                  n137 = Bundle("Number of Disparity"=w343, "Number of Disparity"=0.0) -> (w340:T20)  [unwired: 1 out]
                  n138 = Add(x=w341, y=w340) -> (x+y=w339:cluster{dbl, dbl})
                  n139 = case shown="假" w347 {
                    tunnel: w353 -> [w361 _]
                    tunnel: w352 -> [w360 _]
                    tunnel: w339 -> [w356 _]
                    frame False {
                      n140 = call "IMAQ Convert Pixel To 3D Coordinates"("Binocular Stereo Session"=w361, "Disparity Image"=w360, "Pixel Coordinates"=w356, "Depth Control"="Depth Control") -> ("Real World 3D Coordinates"=w359:cluster{"X":dbl, "Y":dbl, "Z":dbl})  [unwired: 4 in, 7 out]
                      n141 = Unbundle By Name(w359) -> ("Z"=→"Depth":dbl)
                    }
                    frame True {
                    }
                  }
                }
                event "Exit": Value Change {
                  # "Dispose of the session and images"
                  n142 = event-data() -> ()  [unwired: 2 out]
                  n143 = call "IMAQ Dispose"("Image"=w366) -> ()  [unwired: 2 in, 4 out]
                  n144 = call "IMAQ Dispose"("Image"=w365) -> ()  [unwired: 2 in, 4 out]
                  n145 = call "IMAQ Dispose"("Image"=w371) -> ()  [unwired: 2 in, 4 out]
                  n146 = call "IMAQ Dispose"("Image"=w370) -> ()  [unwired: 2 in, 4 out]
                  n147 = call "IMAQ Dispose"("Image"=w369) -> ()  [unwired: 2 in, 4 out]
                  n148 = call "IMAQ Dispose"("Image"=w368) -> ()  [unwired: 2 in, 4 out]
                  n149 = call "IMAQ Dispose"("Image"=w372) -> ()  [unwired: 2 in, 4 out]
                  n150 = call "IMAQ Dispose"("Image"=w367) -> ()  [unwired: 2 in, 4 out]
                  n151 = call "IMAQ Dispose Binocular Stereo Session"("Binocular Stereo Session"=w364) -> ()  [unwired: 1 in, 10 out]
                  n152 = call "IMAQ Dispose"("Image"=w363) -> ()  [unwired: 2 in, 4 out]
                  n153 = call "IMAQ Dispose"("Image"=w362) -> ()  [unwired: 2 in, 4 out]
                }
              }
            }
          }
        }
      }
    }
  }
  n154 = Create User Event(user event datatype=w8) -> (user event=w1:refnum<user-event>)  [unwired: 1 in, 1 out]
  n155 = while {
    tunnel: w1 -> [w390]
    tunnel: [w389] -> w2
    stop <- "stop 2" stop-if-true
    n156 = flat-sequence {
      tunnel: [w397] -> w388
      tunnel: [w398] -> w387
      tunnel: [w397] -> w381
      tunnel: w387 -> [w413]
      tunnel: [w413] -> w386
      tunnel: [w412] -> w382
      tunnel: w381 -> [w412]
      tunnel: [w411] -> w378
      tunnel: w386 -> [w431]
      tunnel: [w431] -> w385
      tunnel: [w430] -> w383
      tunnel: w382 -> [w430]
      tunnel: [w429] -> w379
      tunnel: w378 -> [w429]
      tunnel: [w426] -> w376
      tunnel: w385 -> [w447]
      tunnel: [w446] -> w384
      tunnel: w383 -> [w446]
      tunnel: [w445] -> w380
      tunnel: w379 -> [w445]
      tunnel: [w444] -> w377
      tunnel: w376 -> [w444]
      tunnel: [w442] -> w375
      tunnel: [w443] -> w374
      tunnel: w384 -> [w463]
      tunnel: w380 -> [w462]
      tunnel: w377 -> [w461]
      tunnel: w375 -> [w460]
      tunnel: w374 -> [w459]
      frame #0 {
        n157 = local write "内部数据数组"(string[] ["无效内部数据", "None", "None", "None", "None", "None", "None", "None", "None"] ("环境数据数组")) -> ()
        n158 = local write "环境数据数组"(string[] ["无效环境数据", "None", "0.000", "0.000", "0.00000", "0.000", "0", "0"] ("环境数据数组")) -> ()
      }
      frame #1 {
        n159 = local read "VISA resource name for Modbus"() -> (w398:refnum<visa-resource-name>)
        n160 = call "modbus.vi"("VISA resource name for Modbus"=w398, "起始地址ADR低位"="0") -> ("read buf"=w399:string, "通信指示"=w407:bool)  [unwired: 1 out]
        n161 = property on="Modbus" class="Bool (严格)"("Value"=w407) -> ()  [unwired: 2 in, 2 out]
        n162 = String To Byte Array(string=w399) -> (unsigned byte array=w406:u8[])
        n163 = Index Array(array=w406, index=3 ("offset (0)")) -> (element=w403:u8)
        n164 = Index Array(array=w406, index=4 ("offset (0)")) -> (element=w400:u8)
        n165 = Multiply(x=w403, y=10 ("offset (0)")) -> (x*y=w401:i32)
        n166 = Add(x=w401, y=w400) -> (x+y=w408:i32)
        n167 = Multiply(x=w408, y=0.1) -> (x*y=w397:dbl)
        "温度计" <- w397
        n168 = property on="温度" class="DigNum (严格)"("Value"=w397) -> ()  [unwired: 2 in, 2 out]
      }
      frame #2 {
        n169 = call "modbus.vi"("VISA resource name for Modbus"=w413, "起始地址ADR低位"="1") -> ("read buf"=w417:string, "通信指示"=w416:bool)  [unwired: 1 out]
        n170 = property on="Modbus" class="Bool (严格)"("Value"=w416) -> ()  [unwired: 2 in, 2 out]
        n171 = String To Byte Array(string=w417) -> (unsigned byte array=w424:u8[])
        n172 = Index Array(array=w424, index=3 ("offset (0)")) -> (element=w421:u8)
        n173 = Index Array(array=w424, index=4 ("offset (0)")) -> (element=w418:u8)
        n174 = Multiply(x=w421, y=10 ("offset (0)")) -> (x*y=w419:i32)
        n175 = Add(x=w419, y=w418) -> (x+y=w414:i32)
        n176 = Multiply(x=w414, y=0.1) -> (x*y=w411:dbl)
        "湿度计" <- w411
        n177 = property on="湿度" class="DigNum (严格)"("Value"=w411) -> ()  [unwired: 2 in, 2 out]
      }
      frame #3 {
        n178 = call "modbus.vi"("VISA resource name for Modbus"=w431, "起始地址ADR低位"="2") -> ("read buf"=w438:string, "通信指示"=w432:bool)  [unwired: 1 out]
        n179 = property on="Modbus" class="Bool (严格)"("Value"=w432) -> ()  [unwired: 2 in, 2 out]
        n180 = String To Byte Array(string=w438) -> (unsigned byte array=w435:u8[])
        n181 = Index Array(array=w435, index=3 ("offset (0)")) -> (element=w440:u8)
        n182 = Index Array(array=w435, index=4 ("offset (0)")) -> (element=w427:u8)
        n183 = Multiply(x=w440, y=1000 ("offset (0)")) -> (x*y=w428:i32)
        n184 = Add(x=w428, y=w427) -> (x+y=w437:i32)
        n185 = Multiply(x=w437, y=0.001) -> (x*y=w426:dbl)
        "气压计" <- w426
        n186 = property on="大气压" class="DigNum (严格)"("Value"=w426) -> ()  [unwired: 2 in, 2 out]
      }
      frame #4 {
        n187 = call "modbus.vi"("VISA resource name for Modbus"=w447, "起始地址ADR低位"="3") -> ("read buf"=w454:string, "通信指示"=w443:bool)  [unwired: 1 out]
        n188 = property on="Modbus" class="Bool (严格)"("Value"=w443) -> ()  [unwired: 2 in, 2 out]
        n189 = String To Byte Array(string=w454) -> (unsigned byte array=w451:u8[])
        n190 = Index Array(array=w451, index=3 ("offset (0)")) -> (element=w457:u8)
        n191 = Index Array(array=w451, index=4 ("offset (0)")) -> (element=w450:u8)
        n192 = Multiply(x=w457, y=10 ("offset (0)")) -> (x*y=w455:i32)
        n193 = Add(x=w455, y=w450) -> (x+y=w453:i32)
        n194 = Multiply(x=w453, y=0.1) -> (x*y=w442:dbl)
        "光度计" <- w442
        n195 = property on="光照强度" class="DigNum (严格)"("Value"=w442) -> ()  [unwired: 2 in, 2 out]
      }
      frame #5 {
        n196 = case shown="真" w459 {
          tunnel: w463 -> [w473 _]
          tunnel: w462 -> [w472 _]
          tunnel: w461 -> [w465 _]
          tunnel: w460 -> [w464 _]
          frame True {
            w478 = 0 ("offset (0)")
            n197 = Get Date/Time In Seconds() -> (seconds since 1Jan1904=w500:timestamp)
            n198 = local read "环境数据数组"() -> (w499:string[])
            n199 = local read "Y轴（时间）"() -> (w467:dbl)
            n200 = local read "环境数据"() -> (w479:dbl[][])
            n201 = Replace Array Subset(array="数组", new element #1=w473, index (row) #1=0 ("offset (0)"), index (col) #1=w478, new element #2=w472, index (row) #2=1 ("offset (0)"), index (col) #2=w478, new element #3=w464, index (row) #3=2 ("offset (0)"), index (col) #3=w478, new element #4=w465, index (row) #4=3 ("offset (0)"), index (col) #4=w478) -> (w471:dbl[][])
            n202 = Format Date/Time String(seconds (now)=w500) -> (date/time string=w490:string)  [unwired: 2 in]
            n203 = Number To Fractional String(number=w473, precision (6)=i16 1) -> (F-format string=w489:string)  [unwired: 2 in]
            n204 = Number To Fractional String(number=w472, precision (6)=i16 1) -> (F-format string=w488:string)  [unwired: 2 in]
            n205 = Number To Fractional String(number=w465, precision (6)=i16 3) -> (F-format string=w487:string)  [unwired: 2 in]
            n206 = Number To Fractional String(number=w464, precision (6)=i16 1) -> (F-format string=w485:string)  [unwired: 2 in]
            n207 = Insert Into Array(array=w479, index (col)=w467, new element=w471) -> (→"环境数据":dbl[][])  [unwired: 1 in]
            n208 = Increment(x=w467) -> (x+1=→"Y轴（时间）":dbl)
            n209 = local read "环境数据显示栏值"() -> (w498:string[][])
            n210 = Replace Array Subset(array=w499, new element #1="环境数据", index #1=0 ("offset (0)"), new element #2=w490, index #2=1 ("offset (0)"), new element #3=w489, index #3=2 ("offset (0)"), new element #4=w488, index #4=3 ("offset (0)"), new element #5=w487, index #5=4 ("offset (0)"), new element #6=w485, index #6=5 ("offset (0)"), new element #7="0", index #7=6 ("offset (0)"), new element #8="0", index #8=7 ("offset (0)")) -> (w497:string[])
            n211 = local write "环境数据数组"(w497) -> ()
            n212 = Insert Into Array(array=w498, index (row)=0 ("offset (0)"), new element=w497) -> (w496:string[][])  [unwired: 1 in]
            n213 = local write "环境数据显示栏值"(w496) -> ()
            n214 = property on="环境数据" class="MCListbox (严格)"("ItemNames"=w496) -> ()  [unwired: 2 in, 2 out]
          }
          frame False {
            n215 = local read "环境数据显示栏值"() -> (w505:string[][])
            n216 = local read "环境数据数组"() -> (w506:string[])
            n217 = Insert Into Array(array=w505, index (row)=0 ("offset (0)"), new element=w506) -> (w508:string[][])  [unwired: 1 in]
            n218 = property on="环境数据" class="MCListbox (严格)"("ItemNames"=w508) -> ()  [unwired: 2 in, 2 out]
            n219 = local write "环境数据显示栏值"(w508) -> ()
          }
        }
      }
      frame #6 {
        n220 = property on="GPS" class="Bool (严格)"() -> ("Value"=w509:bool)  [unwired: 2 in, 2 out]
        n221 = case shown="真" w509 {
          frame False {
          }
          frame True {
            n222 = local read "经度"() -> (w518:string)
            n223 = local read "纬度"() -> (w517:string)
            n224 = local read "内部数据数组"() -> (w514:string[])
            n225 = Get Date/Time In Seconds() -> (seconds since 1Jan1904=w523:timestamp)
            n226 = local read "内部数据显示栏值"() -> (w511:string[][])
            n227 = Format Date/Time String(seconds (now)=w523) -> (date/time string=w516:string)  [unwired: 2 in]
            n228 = Replace Array Subset(array=w514, new element #1=w516, index #1=0 ("offset (0)"), new element #2="内部数据", index #2=1 ("offset (0)"), new element #3=w518, index #3=5 ("offset (0)"), new element #4=w517, index #4=6 ("offset (0)")) -> (w512:string[])
            n229 = Insert Into Array(array=w511, index (row)=0 ("offset (0)"), new element=w512) -> (w510:string[][])  [unwired: 1 in]
            n230 = local write "内部数据数组"(w512) -> ()
            n231 = property on="内部数据" class="MCListbox (严格)"("ItemNames"=w510) -> ()  [unwired: 2 in, 2 out]
            n232 = local write "内部数据显示栏值"(w510) -> ()
          }
        }
      }
    }
    n233 = Wait (ms)(milliseconds to wait=u32 5000) -> ()  [unwired: 1 out]
    n234 = Greater?(x=w388, y="报警上限") -> (0:w391:bool)
    "发生报警" <- w391
    n235 = case shown="真" w391 {
      tunnel: w390 -> [_ w526]
      tunnel: w388 -> [_ w525]
      tunnel: [_ w524] -> w389
      frame False {
      }
      frame True {
        n236 = Generate User Event(user event=w526, event data cluster=w525) -> (error out=w524:errorcluster)  [unwired: 1 in, 1 out]
      }
    }
  }
  n237 = register-events(w1) -> (reference out=w7:refnum<event-registration>)  [unwired: 2 in, 1 out]
  n238 = while {
    shift-right: [w532] -> _
    shift-left: w4 -> [w533]
    tunnel: w7 -> [w531]
    shift-right: [w529] -> _
    shift-left: w6 -> [w530]
    tunnel: [w528] -> w5
    stop <- w527 stop-if-true
    n239 = event shown="[0] <温度报警>: 用户事件" {
      selector: w531 -> [_ _ _]
      dyn-events: [_ _ _] -> w528
      timeout: _ -> [_ _ _]
      tunnel: w533 -> [w538 _ _]
      tunnel: [w534 _ _] -> w532
      tunnel: w530 -> [w544 _ _]
      tunnel: [w537 _ _] -> w529
      tunnel: [_ _ w547] -> w527
      event User Event {
        n240 = event-data() -> ("温度报警"=w540:dbl)  [unwired: 1 in]
        n241 = Increment(x=w538) -> (x+1=w534:i32)
        n242 = Get Date/Time In Seconds() -> (seconds since 1Jan1904=w536:timestamp)
        n243 = local write "报警数"(w534) -> ()
        n244 = Format Date/Time String(seconds (now)=w536) -> (date/time string=w543:string)  [unwired: 2 in]
        n245 = Number To Decimal String(number=w534) -> (decimal integer string=w542:string)  [unwired: 1 in]
        n246 = Number To Fractional String(number=w540, precision (6)=i16 3) -> (F-format string=w539:string)  [unwired: 2 in]
        n247 = Build Array(w542, w543, w539) -> (w541:string[])
        n248 = Build Array (concatenate)(w544, w541) -> (w537:string[][])
        n249 = local write "报警历史"(w537) -> ()
      }
      event "清除报警": Value Change {
        n250 = event-data() -> ()  [unwired: 1 in, 2 out]
        n251 = local write "报警数"(0 ("报警数")) -> ()
        n252 = local write "报警历史"(string[][] [] ("报警历史")) -> ()
      }
      event "stop 2": Value Change {
        n253 = event-data() -> ("NewVal"=w547:bool)  [unwired: 1 in]
      }
    }
  }
  n254 = while {
    tunnel: w12 -> [w581]
    tunnel: w11 -> [w582]
    tunnel: [w589] -> w13
    tunnel: [w590] -> w14
    tunnel: w10 -> [w580]
    tunnel: "颜色簇" -> [w558]
    stop <- "stop" stop-if-true
    n255 = local read "经度"() -> (w553:string)
    n256 = local read "纬度"() -> (w552:string)
    n257 = VISA Read(VISA resource name=w581, byte count=w580, error in (no error)=w582) -> (VISA resource name out=w590:refnum<visa-resource-name>, read buffer=w584:string, error out=w589:errorcluster)  [unwired: 1 out]
    "actual data" <- w584
    n258 = Get Date/Time String() -> (date string=→"日期字符串":string, time string=→"时间字符串":string)  [unwired: 3 in]
    n259 = Get Date/Time In Seconds() -> (seconds since 1Jan1904=→"时间标识":timestamp)
    n260 = event shown="[1] \"生成报表\": 值改变" {
      selector: _ -> [_ _ _ _]
      dyn-events: _ -> [_ _ _ _]
      timeout: 1 -> [_ _ _ _]
      event "当前报警": Double Click {
        n261 = event-data() -> ("Row"=w591:i32)  [unwired: 1 in, 7 out]
        n262 = local read "数据显示栏值"() -> (w596:string[][])
        n263 = local read "时间字符串"() -> (w592:string)
        n264 = local read "报警没确认行号数组"() -> (w603:dbl[])
        n265 = Add(x=w591, y=1) -> (x+y=w604:i32)
        n266 = local read "报警已确认行号数组"() -> (w597:dbl[])
        n267 = local read "报警没确认行号数组"() -> (w599:dbl[])
        n268 = Replace Array Subset(array=w596, new element=w592, index (row)=w591, index (col)=3 ("禁用的索引 (列)")) -> (w595:string[][])
        n269 = Search 1D Array(1D array=w603, element=w604) -> (index of element=w594:i32)  [unwired: 1 in]
        n270 = local write "数据显示栏值"(w595) -> ()
        n271 = Index Array(array=w599, index=w594) -> (element=w600:dbl)
        n272 = Array Size(array=w597) -> (size(s)=w598:i32)
        n273 = Delete From Array(array=w603, index=w594) -> (array with subset deleted=w602:dbl[])  [unwired: 1 in, 1 out]
        n274 = local write "报警没确认行号数组"(w602) -> ()
        n275 = Insert Into Array(array=w597, index=w598, new element=w600) -> (w601:dbl[])
        n276 = local write "报警已确认行号数组"(w601) -> ()
      }
      event "生成报表": Value Change {
        n277 = event-data() -> ()  [unwired: 1 in, 5 out]
        n278 = local read "日期字符串"() -> (w610:string)
        n279 = local read "时间字符串"() -> (w608:string)
        n280 = Concatenate Strings("日期:", w610, " 时间:", w608) -> (w609:string)
        n281 = local read "数据显示栏值"() -> (w615:string[][])
        n282 = Unbundle By Name("表格") -> ("auto format"=w618:i32, "font"=w617:T4)  [unwired: 1 out]
        n283 = Unbundle By Name("报表信息") -> ("font"=w612:T4)  [unwired: 1 out]
        n284 = Bundle By Name(cluster="表格", "auto format"=w618, "font"=w617, "表格 2"=w615) -> (w616:T5)
        n285 = Bundle By Name(cluster="报表信息", "font"=w612, "字符串"=w609) -> (w611:cluster{"font":T4, "字符串":string})
        n286 = local read "当前报警"() -> (w614:i32)
        n287 = call "Html Report.vi"("报表信息"=w611, "表格"=w616, "当前报警"=w614) -> ()  [unwired: 17 in]
      }
      event "写入数据库": Value Change {
        n288 = event-data() -> ()  [unwired: 1 in, 5 out]
        n289 = property on="数据显示栏值" class="Arr (严格)"() -> ("Number of Rows"=w620:u32)  [unwired: 2 in, 2 out]
        n290 = for {
          N: w620 -> [_]
          i -> [w649]
          n291 = local read "数据显示栏值"() -> (w648:string[][])
          n292 = Index Array(array=w648, index (row)=w649) -> (element=w629:string[])  [unwired: 1 in]
          n293 = Index Array(array=w629, index=9) -> (element=w624:string)
          n294 = Index Array(array=w629, index=8) -> (element=w626:string)
          n295 = Index Array(array=w629, index=6) -> (element=w636:string)
          n296 = Index Array(array=w629, index=5) -> (element=w637:string)
          n297 = Index Array(array=w629, index=1) -> (element=w646:string)
          n298 = Index Array(array=w629, index=2) -> (element=w640:string)
          n299 = Index Array(array=w629, index=3) -> (element=w639:string)
          n300 = Index Array(array=w629, index=4) -> (element=w638:string)
          n301 = Index Array(array=w629, index=7) -> (element=w630:string)
          n302 = Index Array(array=w629, index=10) -> (element=w627:string)
          n303 = Index Array(array=w629, index=11) -> (element=w621:string)
          n304 = Decimal String To Number(string=w624) -> (number=w623:i32)  [unwired: 2 in, 1 out]
          n305 = Decimal String To Number(string=w626) -> (number=w625:i32)  [unwired: 2 in, 1 out]
          n306 = Decimal String To Number(string=w627) -> (number=w628:i32)  [unwired: 2 in, 1 out]
          n307 = Decimal String To Number(string=w621) -> (number=w622:i32)  [unwired: 2 in, 1 out]
          n308 = call "AlarmTable.vi"("HH值"=w622, "H值"=w628, "L值"=w623, "LL值"=w625, "报警值"=w636, "单位"=w630, "报警形式"=w637, "消除时间"=w638, "确认时间"=w639, "报警时间"=w640, "名称"=w646) -> ()  [unwired: 1 out]
        }
      }
      event Timeout {
        n309 = event-data() -> ()  [unwired: 1 in, 2 out]
      }
    }
    n310 = Unbundle By Name(w558) -> ("报警没确认"=w565:u32, "背景色"=w562:u32, "消除没确认"=w564:u32, "报警已确认"=w563:u32)
    n311 = event shown="[4] \"测试图片\": 值改变" {
      selector: _ -> [_ _ _ _ _ _]
      dyn-events: _ -> [_ _ _ _ _ _]
      timeout: 1 ("y") -> [_ _ _ _ _ _]
      event Timeout {
        n312 = event-data() -> ()  [unwired: 1 in, 2 out]
      }
      event "运行状态.小车状态": Value Change {
        n313 = event-data() -> ("NewVal"=w704:bool)  [unwired: 1 in, 4 out]
        n314 = case shown="真" w704 {
          frame False {
            n315 = local read "时间字符串"() -> (w705:string)
            n316 = property on="停止时间" class="Str"("Value"=w705) -> ()  [unwired: 2 in, 2 out]
          }
          frame True {
            n317 = local read "时间字符串"() -> (w706:string)
            n318 = property on="开始时间" class="Str"("Value"=w706) -> ()  [unwired: 2 in, 2 out]
          }
        }
      }
      event "确定按钮": Value Change {
        n319 = event-data() -> ()  [unwired: 1 in, 5 out]
        n320 = call "modbus.vi"("VISA resource name for Modbus"="VISA resource name for Modbus", "起始地址ADR低位"="从机数据地址") -> ("read buf"=w716:string, "通信指示"=w718:bool)  [unwired: 1 out]
        "Modbus报文" <- w716
        n321 = property on="Modbus" class="Bool (严格)"("Value"=w718) -> ()  [unwired: 2 in, 2 out]
        n322 = String To Byte Array(string=w716) -> (unsigned byte array=w715:u8[])
        n323 = Index Array(array=w715, index=3 ("offset (0)")) -> (element=w712:u8)
        n324 = Index Array(array=w715, index=4 ("offset (0)")) -> (element=w709:u8)
        n325 = Multiply(x=w712, y=10 ("offset (0)")) -> (x*y=w710:i32)
        n326 = Add(x=w710, y=w709) -> (x+y=→"值":i32)
      }
      event "stop": Value Change {
        n327 = event-data() -> ()  [unwired: 1 in, 5 out]
        n328 = Stop() -> ()  [unwired: 1 in]
      }
      event "测试图片": Value Change {
        n329 = event-data() -> ("NewVal"=w719:i8)  [unwired: 1 in, 4 out]
        n330 = Greater?(x=w719, y=0) -> (0:w721:bool)
        n331 = flat-sequence {
          tunnel: w721 -> [w723]
          tunnel: w719 -> [w722]
          frame #0 {
            n332 = case shown="真" w723 {
              tunnel: w722 -> [_ w730]
              frame False {
                w724 = 0
                n333 = local write "果实"(w724) -> ()
                n334 = local write "花朵"(w724) -> ()
                n335 = local write "花蕾"(w724) -> ()
                n336 = local write "正常叶片"(w724) -> ()
                n337 = local write "问题叶片"(w724) -> ()
                n338 = local write "未成熟果实"(w724) -> ()
              }
              frame True {
                n339 = Current VI's Path() -> (path=w729:path)
                n340 = Number To Decimal String(number=w730) -> (decimal integer string=w733:string)  [unwired: 1 in]
                n341 = Path To String(path=w729) -> (string=w728:string)
                n342 = Search and Replace String(input string=w728, search string="main.vi", replace string="测试图片") -> (result string=w725:string)  [unwired: 5 in, 3 out]
                n343 = Concatenate Strings(w733, ".jpg" ("name or relative path")) -> (w731:string)
                n344 = String To Path(string=w725) -> (path=w743:path)
                n345 = Build Path(base path=w743, name or relative path=w731) -> (appended path=w742:path)
                n346 = local read "主摄像头"() -> (w741:T8)
                n347 = call "IMAQ ReadFile"("File Path"=w742, "Image"=w741) -> ("Image Out"=w735:T8)  [unwired: 3 in, 6 out]
                n348 = local write "主摄像头"(w735) -> ()
                n349 = call "TroubleLeaf.vi"("Image In"=w735) -> ("Number of Matches (TroubleLeaf)"=w734:i32)  [unwired: 22 in, 4 out]
                n350 = call "RipeFruit.vi"("Image In"=w735) -> ("Number of Matches (RipeFruit)"=w740:i32)  [unwired: 22 in, 4 out]
                n351 = call "flower.vi"("Image In"=w735) -> ("Number of Matches (Color Pattern Matching 1)"=w738:i32)  [unwired: 22 in, 4 out]
                n352 = call "Leaf.vi"("Image In"=w735) -> ("Number of Matches (Leaf)"=w736:i32)  [unwired: 22 in, 4 out]
                n353 = call "Bud.vi"("Image In"=w735) -> ("Number of Matches (Bud)"=w737:i32)  [unwired: 22 in, 4 out]
                n354 = call "NotRipeFruit.vi"("Image In"=w735) -> ("Number of Matches (NotRipeFruit)"=w739:i32)  [unwired: 22 in, 4 out]
                n355 = local write "问题叶片"(w734) -> ()
                n356 = local write "果实"(w740) -> ()
                n357 = local write "花朵"(w738) -> ()
                n358 = local write "正常叶片"(w736) -> ()
                n359 = local write "花蕾"(w737) -> ()
                n360 = local write "未成熟果实"(w739) -> ()
              }
            }
          }
          frame #1 {
            n361 = property on="当前报警列表框" class="MCListbox (严格)"() -> ("NumRows"=w744:u32)  [unwired: 2 in, 2 out]
            n362 = for {
              N: w744 -> [_]
              i -> [w753]
              n363 = control-ref of="报警设置"() -> (w754:refnum<vi>)
              n364 = property on="属性节点" class="MCListbox (严格)"(reference=w754) -> ("ItemNames"=w751:string[][])  [unwired: 1 in, 2 out]
              n365 = Index Array(array=w751, index (row)=w753) -> (element=w745:string[])  [unwired: 1 in]
              n366 = Search 1D Array(1D array=w745, element="果实") -> (index of element=w748:i32)  [unwired: 1 in]
              n367 = Search 1D Array(1D array=w745, element="问题叶片") -> (index of element=w750:i32)  [unwired: 1 in]
              n368 = Greater Than 0?(x=w750) -> (x > 0?=w749:bool)
              n369 = Greater Than 0?(x=w748) -> (x > 0?=w746:bool)
              n370 = case shown="真" w749 {
                tunnel: w745 -> [_ w841]
                frame False {
                }
                frame True {
                  n371 = Index Array(array=w841, index=11) -> (element=w850:string)
                  n372 = Index Array(array=w841, index=10) -> (element=w849:string)
                  n373 = Index Array(array=w841, index=9) -> (element=w848:string)
                  n374 = Index Array(array=w841, index=8) -> (element=w851:string)
                  n375 = local read "问题叶片"() -> (w847:dbl)
                  n376 = Decimal String To Number(string=w850) -> (number=w843:i32)  [unwired: 2 in, 1 out]
                  n377 = Decimal String To Number(string=w849) -> (number=w844:i32)  [unwired: 2 in, 1 out]
                  n378 = Decimal String To Number(string=w848) -> (number=w845:i32)  [unwired: 2 in, 1 out]
                  n379 = Decimal String To Number(string=w851) -> (number=w846:i32)  [unwired: 2 in, 1 out]
                  n380 = formula code="if(i<LL)\nOut=0;\nelse if(i>=LL&&i<L)\nOut=1;\nelse if(i>=L&&i<H)\nOut=2;\nelse if(i>=H&&i<HH)\nOut=3;\nelse if(i>=HH)\nOut=4;"("i"=w847, "HH"=w843, "H"=w844, "L"=w845, "LL"=w846) -> ("Out"=w842:dbl)
                  n381 = flat-sequence {
                    tunnel: w842 -> [w861]
                    tunnel: [w861] -> w840
                    tunnel: w840 -> [w862]
                    frame #0 {
                      n382 = local read "问题叶片"() -> (w859:dbl)
                      n383 = local read "问题叶片报警数组"() -> (w860:string[])
                      n384 = Number To Decimal String(number=w859) -> (decimal integer string=w857:string)  [unwired: 1 in]
                      n385 = Replace Array Subset(array=w860, new element=w857, index=6) -> (w858:string[])
                      n386 = local write "问题叶片报警数组"(w858) -> ()
                    }
                    frame #1 {
                      n387 = case shown="4" w862 {
                        frame 0, Default {
                          n388 = local read "问题叶片报警数组"() -> (w871:string[])
                          n389 = local write "问题叶片"(TRUE ("问题叶片")) -> ()
                          n390 = local read "时间字符串"() -> (w872:string)
                          n391 = local read "数据显示栏值"() -> (w869:string[][])
                          n392 = local read "报警没确认行号数组"() -> (w865:dbl[])
                          n393 = local read "报警计数"() -> (w864:dbl)
                          n394 = Replace Array Subset(array=w871, new element #1="LL报警", index #1=5, new element #2=w872, index #2=2) -> (w868:string[])
                          n395 = Insert Into Array(array=w869, index (row)=w864, new element=w868) -> (w870:string[][])  [unwired: 1 in]
                          n396 = local write "问题叶片报警数组"(w868) -> ()
                          n397 = Increment(x=w864) -> (x+1=w867:dbl)
                          n398 = local write "数据显示栏值"(w870) -> ()
                          n399 = Insert Into Array(array=w865, new element=w867) -> (w866:dbl[])  [unwired: 1 in]
                          n400 = local write "报警计数"(w867) -> ()
                          n401 = local write "报警没确认行号数组"(w866) -> ()
                        }
                        frame 1 {
                          n402 = local read "问题叶片报警数组"() -> (w884:string[])
                          n403 = local write "问题叶片"(TRUE ("问题叶片")) -> ()
                          n404 = local read "时间字符串"() -> (w885:string)
                          n405 = local read "数据显示栏值"() -> (w882:string[][])
                          n406 = local read "报警没确认行号数组"() -> (w878:dbl[])
                          n407 = local read "报警计数"() -> (w877:dbl)
                          n408 = Replace Array Subset(array=w884, new element #1="L报警", index #1=5, new element #2=w885, index #2=2) -> (w881:string[])
                          n409 = Insert Into Array(array=w882, index (row)=w877, new element=w881) -> (w883:string[][])  [unwired: 1 in]
                          n410 = local write "问题叶片报警数组"(w881) -> ()
                          n411 = Increment(x=w877) -> (x+1=w880:dbl)
                          n412 = local write "数据显示栏值"(w883) -> ()
                          n413 = Insert Into Array(array=w878, new element=w880) -> (w879:dbl[])  [unwired: 1 in]
                          n414 = local write "报警计数"(w880) -> ()
                          n415 = local write "报警没确认行号数组"(w879) -> ()
                        }
                        frame 2 {
                          n416 = disable-structure shown="禁用" {
                            frame Disabled {
                              n417 = local read "问题叶片报警数组"() -> (w894:string[])
                              n418 = local read "时间字符串"() -> (w895:string)
                              n419 = local read "数据显示栏值"() -> (w892:string[][])
                              n420 = local read "报警计数"() -> (w890:dbl)
                              n421 = Replace Array Subset(array=w894, new element #1="正常", index #1=5, new element #2=w895, index #2=2) -> (w891:string[])
                              n422 = Insert Into Array(array=w892, index (row)=w890, new element=w891) -> (w893:string[][])  [unwired: 1 in]
                              n423 = local write "问题叶片报警数组"(w891) -> ()
                              n424 = local write "数据显示栏值"(w893) -> ()
                            }
                            frame Enabled {
                            }
                          }
                          n425 = local write "问题叶片"(FALSE ("问题叶片")) -> ()
                        }
                        frame 3 {
                          n426 = local read "问题叶片报警数组"() -> (w907:string[])
                          n427 = local write "问题叶片"(TRUE ("问题叶片")) -> ()
                          n428 = local read "时间字符串"() -> (w908:string)
                          n429 = local read "数据显示栏值"() -> (w905:string[][])
                          n430 = local read "报警没确认行号数组"() -> (w901:dbl[])
                          n431 = local read "报警计数"() -> (w900:dbl)
                          n432 = Replace Array Subset(array=w907, new element #1="H报警", index #1=5, new element #2=w908, index #2=2) -> (w904:string[])
                          n433 = Insert Into Array(array=w905, index (row)=w900, new element=w904) -> (w906:string[][])  [unwired: 1 in]
                          n434 = local write "问题叶片报警数组"(w904) -> ()
                          n435 = Increment(x=w900) -> (x+1=w903:dbl)
                          n436 = local write "数据显示栏值"(w906) -> ()
                          n437 = Insert Into Array(array=w901, new element=w903) -> (w902:dbl[])  [unwired: 1 in]
                          n438 = local write "报警计数"(w903) -> ()
                          n439 = local write "报警没确认行号数组"(w902) -> ()
                        }
                        frame 4 {
                          n440 = local read "问题叶片报警数组"() -> (w920:string[])
                          n441 = local write "问题叶片"(TRUE ("问题叶片")) -> ()
                          n442 = local read "时间字符串"() -> (w921:string)
                          n443 = local read "数据显示栏值"() -> (w918:string[][])
                          n444 = local read "报警没确认行号数组"() -> (w914:dbl[])
                          n445 = local read "报警计数"() -> (w913:dbl)
                          n446 = Replace Array Subset(array=w920, new element #1="HH报警", index #1=5, new element #2=w921, index #2=2) -> (w917:string[])
                          n447 = Insert Into Array(array=w918, index (row)=w913, new element=w917) -> (w919:string[][])  [unwired: 1 in]
                          n448 = local write "问题叶片报警数组"(w917) -> ()
                          n449 = Increment(x=w913) -> (x+1=w916:dbl)
                          n450 = local write "数据显示栏值"(w919) -> ()
                          n451 = Insert Into Array(array=w914, new element=w916) -> (w915:dbl[])  [unwired: 1 in]
                          n452 = local write "报警计数"(w916) -> ()
                          n453 = local write "报警没确认行号数组"(w915) -> ()
                        }
                      }
                    }
                  }
                  "问题叶片报警数组" <- w841
                }
              }
              n454 = case shown="真" w746 {
                tunnel: w745 -> [_ w757]
                frame False {
                }
                frame True {
                  n455 = Index Array(array=w757, index=11) -> (element=w765:string)
                  n456 = Index Array(array=w757, index=10) -> (element=w764:string)
                  n457 = Index Array(array=w757, index=9) -> (element=w763:string)
                  n458 = Index Array(array=w757, index=8) -> (element=w766:string)
                  n459 = Decimal String To Number(string=w765) -> (number=w759:i32)  [unwired: 2 in, 1 out]
                  n460 = Decimal String To Number(string=w764) -> (number=w760:i32)  [unwired: 2 in, 1 out]
                  n461 = Decimal String To Number(string=w763) -> (number=w761:i32)  [unwired: 2 in, 1 out]
                  n462 = Decimal String To Number(string=w766) -> (number=w762:i32)  [unwired: 2 in, 1 out]
                  n463 = local read "果实"() -> (w756:dbl)
                  n464 = formula code="if(i<LL)\nOut=0;\nelse if(i>=LL&&i<L)\nOut=1;\nelse if(i>=L&&i<H)\nOut=2;\nelse if(i>=H&&i<HH)\nOut=3;\nelse if(i>=HH)\nOut=4;"("i"=w756, "HH"=w759, "H"=w760, "L"=w761, "LL"=w762) -> ("Out"=w758:dbl)
                  n465 = flat-sequence {
                    tunnel: w758 -> [w776]
                    tunnel: [w776] -> w755
                    tunnel: w755 -> [w777]
                    frame #0 {
                      n466 = local read "果实报警数组"() -> (w775:string[])
                      n467 = local read "果实"() -> (w773:dbl)
                      n468 = Number To Decimal String(number=w773) -> (decimal integer string=w772:string)  [unwired: 1 in]
                      n469 = Replace Array Subset(array=w775, new element=w772, index=6) -> (w771:string[])
                      n470 = local write "果实报警数组"(w771) -> ()
                    }
                    frame #1 {
                      n471 = case shown="4" w777 {
                        frame 0, Default {
                          n472 = local write "果实"(TRUE) -> ()
                          n473 = local read "果实报警数组"() -> (w786:string[])
                          n474 = local read "时间字符串"() -> (w787:string)
                          n475 = local read "数据显示栏值"() -> (w784:string[][])
                          n476 = local read "报警没确认行号数组"() -> (w782:dbl[])
                          n477 = local read "报警计数"() -> (w779:dbl)
                          n478 = Replace Array Subset(array=w786, new element #1="LL报警", index #1=5, new element #2=w787, index #2=2) -> (w783:string[])
                          n479 = Insert Into Array(array=w784, index (row)=w779, new element=w783) -> (w785:string[][])  [unwired: 1 in]
                          n480 = local write "果实报警数组"(w783) -> ()
                          n481 = Increment(x=w779) -> (x+1=w780:dbl)
                          n482 = local write "数据显示栏值"(w785) -> ()
                          n483 = local write "报警计数"(w780) -> ()
                          n484 = Insert Into Array(array=w782, new element=w780) -> (w781:dbl[])  [unwired: 1 in]
                          n485 = local write "报警没确认行号数组"(w781) -> ()
                        }
                        frame 1 {
                          n486 = local write "果实"(TRUE) -> ()
                          n487 = local read "果实报警数组"() -> (w799:string[])
                          n488 = local read "时间字符串"() -> (w800:string)
                          n489 = local read "数据显示栏值"() -> (w797:string[][])
                          n490 = local read "报警没确认行号数组"() -> (w795:dbl[])
                          n491 = local read "报警计数"() -> (w792:dbl)
                          n492 = Replace Array Subset(array=w799, new element #1="L报警", index #1=5, new element #2=w800, index #2=2) -> (w796:string[])
                          n493 = Insert Into Array(array=w797, index (row)=w792, new element=w796) -> (w798:string[][])  [unwired: 1 in]
                          n494 = local write "果实报警数组"(w796) -> ()
                          n495 = Increment(x=w792) -> (x+1=w793:dbl)
                          n496 = local write "数据显示栏值"(w798) -> ()
                          n497 = local write "报警计数"(w793) -> ()
                          n498 = Insert Into Array(array=w795, new element=w793) -> (w794:dbl[])  [unwired: 1 in]
                          n499 = local write "报警没确认行号数组"(w794) -> ()
                        }
                        frame 2 {
                          n500 = disable-structure shown="禁用" {
                            frame Disabled {
                              n501 = local read "果实报警数组"() -> (w809:string[])
                              n502 = local read "时间字符串"() -> (w810:string)
                              n503 = local read "数据显示栏值"() -> (w807:string[][])
                              n504 = local read "报警计数"() -> (w805:dbl)
                              n505 = Replace Array Subset(array=w809, new element #1="正常", index #1=5, new element #2=w810, index #2=2) -> (w806:string[])
                              n506 = local write "果实报警数组"(w806) -> ()
                              n507 = Insert Into Array(array=w807, index (row)=w805, new element=w806) -> (w808:string[][])  [unwired: 1 in]
                              n508 = local write "数据显示栏值"(w808) -> ()
                            }
                            frame Enabled {
                            }
                          }
                          n509 = local write "果实"(FALSE ("果实")) -> ()
                        }
                        frame 3 {
                          n510 = local write "果实"(TRUE) -> ()
                          n511 = local read "果实报警数组"() -> (w822:string[])
                          n512 = local read "时间字符串"() -> (w823:string)
                          n513 = local read "数据显示栏值"() -> (w820:string[][])
                          n514 = local read "报警没确认行号数组"() -> (w818:dbl[])
                          n515 = local read "报警计数"() -> (w815:dbl)
                          n516 = Replace Array Subset(array=w822, new element #1="H报警", index #1=5, new element #2=w823, index #2=2) -> (w819:string[])
                          n517 = Insert Into Array(array=w820, index (row)=w815, new element=w819) -> (w821:string[][])  [unwired: 1 in]
                          n518 = local write "果实报警数组"(w819) -> ()
                          n519 = Increment(x=w815) -> (x+1=w816:dbl)
                          n520 = local write "数据显示栏值"(w821) -> ()
                          n521 = local write "报警计数"(w816) -> ()
                          n522 = Insert Into Array(array=w818, new element=w816) -> (w817:dbl[])  [unwired: 1 in]
                          n523 = local write "报警没确认行号数组"(w817) -> ()
                        }
                        frame 4 {
                          n524 = local write "果实"(TRUE) -> ()
                          n525 = local read "果实报警数组"() -> (w835:string[])
                          n526 = local read "时间字符串"() -> (w836:string)
                          n527 = local read "数据显示栏值"() -> (w833:string[][])
                          n528 = local read "报警没确认行号数组"() -> (w831:dbl[])
                          n529 = local read "报警计数"() -> (w828:dbl)
                          n530 = Replace Array Subset(array=w835, new element #1="HH报警", index #1=5, new element #2=w836, index #2=2) -> (w832:string[])
                          n531 = Insert Into Array(array=w833, index (row)=w828, new element=w832) -> (w834:string[][])  [unwired: 1 in]
                          n532 = local write "果实报警数组"(w832) -> ()
                          n533 = Increment(x=w828) -> (x+1=w829:dbl)
                          n534 = local write "数据显示栏值"(w834) -> ()
                          n535 = local write "报警计数"(w829) -> ()
                          n536 = Insert Into Array(array=w831, new element=w829) -> (w830:dbl[])  [unwired: 1 in]
                          n537 = local write "报警没确认行号数组"(w830) -> ()
                        }
                      }
                    }
                  }
                  "果实报警数组" <- w757
                }
              }
            }
          }
          frame #2 {
            n538 = local read "数据显示栏值"() -> (w926:string[][])
            n539 = control-ref of="当前报警列表框"() -> (w925:refnum<vi>)
            n540 = property on="属性节点" class="MCListbox (严格)"(reference=w925, "ItemNames"=w926) -> ()  [unwired: 1 in, 2 out]
          }
        }
      }
      event "Clean": Value Change {
        n541 = event-data() -> ()  [unwired: 1 in, 5 out]
        n542 = flat-sequence {
          frame #0 {
            n543 = local read "报警没确认行号数组"() -> (w927:dbl[])
            n544 = local write "消除未确认行号数组"(w927) -> ()
          }
          frame #1 {
            n545 = property on="报警没确认行号数组" class="Arr (严格)"() -> ("Number of Rows"=w928:u32)  [unwired: 2 in, 2 out]
            n546 = for {
              N: w928 -> [_]
              i -> [w933]
              n547 = local read "报警没确认行号数组"() -> (w934:dbl[])
              n548 = local read "数据显示栏值"() -> (w935:string[][])
              n549 = Index Array(array=w934, index=w933) -> (element=w932:dbl)
              n550 = local read "时间字符串"() -> (w929:string)
              n551 = Replace Array Subset(array=w935, new element=w929, index (row)=w932, index (col)=4 ("禁用的索引 (列)")) -> (w930:string[][])
              n552 = local write "数据显示栏值"(w930) -> ()
            }
          }
          frame #2 {
            n553 = local read "报警没确认行号数组"() -> (w938:dbl[])
            n554 = property on="报警没确认行号数组" class="Arr (严格)"() -> ("Number of Rows"=w936:u32)  [unwired: 2 in, 2 out]
            n555 = Delete From Array(array=w938, length=w936) -> (array with subset deleted=w937:dbl[])  [unwired: 1 in, 1 out]
            n556 = local write "报警没确认行号数组"(w937) -> ()
          }
        }
      }
    }
    n557 = control-ref of="当前报警"() -> (w559:refnum<vi>)
    n558 = property on="数据显示栏值" class="Arr (严格)"() -> ("Number of Rows"=w560:u32)  [unwired: 2 in, 2 out]
    n559 = local read "测试图片"() -> (w549:i8)
    n560 = local read "当前报警"() -> (→"报警设置":i32)
    n561 = local read "UTC时间"() -> (w573:string)
    n562 = local read "主摄像头开关"() -> (w551:bool)
    n563 = Fract/Exp String To Number(string=w553) -> (number=w555:dbl)  [unwired: 3 in, 1 out]
    n564 = Fract/Exp String To Number(string=w552) -> (number=w554:dbl)  [unwired: 3 in, 1 out]
    n565 = property on="主摄像头" class="ImageControl"() -> ("Image Information String"=w569:string)  [unwired: 2 in, 2 out]
    n566 = Equal To 0?(x=w549) -> (x = 0?=w548:bool)
    n567 = for {
      N: w560 -> [_]
      tunnel: w565 -> [w666]
      tunnel: w563 -> [w665]
      tunnel: w564 -> [w659]
      tunnel: w562 -> [w657]
      tunnel: w559 -> [w650]
      i -> [w658]
      n568 = local read "消除未确认行号数组"() -> (w661:dbl[])
      n569 = local read "报警已确认行号数组"() -> (w671:dbl[])
      n570 = local read "报警没确认行号数组"() -> (w676:dbl[])
      n571 = Add(x=w658, y=1) -> (x+y=w662:i32)
      n572 = Add(x=w658, y=1) -> (x+y=w667:i32)
      n573 = Add(x=w658, y=1) -> (x+y=w672:i32)
      n574 = Search 1D Array(1D array=w661, element=w662) -> (index of element=w656:i32)  [unwired: 1 in]
      n575 = Search 1D Array(1D array=w671, element=w667) -> (index of element=w655:i32)  [unwired: 1 in]
      n576 = Search 1D Array(1D array=w676, element=w672) -> (index of element=w654:i32)  [unwired: 1 in]
      n577 = formula code="int16 y;\nif((x1==-1)&&(x2==-1)&&(x3==-1))\n{\ny=-1;\n}\nelse\n{\ny=0;\n}"("x1"=w656, "x2"=w655, "x3"=w654) -> ("y"=w652:i16)
      n578 = Not Equal?(x=w656, y=-1) -> (x != y?=w660:bool)
      n579 = Not Equal?(x=w655, y=-1) -> (x != y?=w669:bool)
      n580 = Not Equal?(x=w654, y=-1) -> (x != y?=w674:bool)
      n581 = case shown="真" w660 {
        tunnel: w658 -> [_ w685]
        tunnel: w659 -> [_ w684]
        tunnel: w650 -> [_ w683]
        frame False {
        }
        frame True {
          n582 = Bundle By Name(cluster=T21 {"Row"=0, "Column"=0} ("活动单元格:活动单元格"), "Row"=w685, "Column"=0) -> (w688:T21)
          n583 = property class="MCListbox (严格)"(reference=w683, "ActiveCell"=w688, "CellBG"=w684) -> ()  [unwired: 1 in, 2 out]
        }
      }
      n584 = case shown="真" w669 {
        tunnel: w658 -> [_ w691]
        tunnel: w665 -> [_ w690]
        tunnel: w650 -> [_ w689]
        frame False {
        }
        frame True {
          n585 = Bundle By Name(cluster=T21 {"Row"=0, "Column"=0} ("活动单元格:活动单元格"), "Row"=w691, "Column"=0) -> (w694:T21)
          n586 = property class="MCListbox (严格)"(reference=w689, "ActiveCell"=w694, "CellBG"=w690) -> ()  [unwired: 1 in, 2 out]
        }
      }
      n587 = case shown="真" w674 {
        tunnel: w658 -> [_ w696]
        tunnel: w650 -> [_ w697]
        tunnel: w666 -> [_ w695]
        frame False {
        }
        frame True {
          n588 = Bundle By Name(cluster=T21 {"Row"=0, "Column"=0} ("活动单元格:活动单元格"), "Row"=w696, "Column"=0) -> (w700:T21)
          n589 = property class="MCListbox (严格)"(reference=w697, "ActiveCell"=w700, "CellBG"=w695) -> ()  [unwired: 1 in, 2 out]
        }
      }
      n590 = Equal?(x=w652, y=-1) -> (x = y?=w651:bool)
      n591 = case shown="真" w651 {
        tunnel: w658 -> [_ w679]
        tunnel: w657 -> [_ w678]
        tunnel: w650 -> [_ w677]
        frame False {
        }
        frame True {
          n592 = Bundle By Name(cluster=T21 {"Row"=0, "Column"=0} ("活动单元格:活动单元格"), "Row"=w679, "Column"=0) -> (w682:T21)
          n593 = property class="MCListbox (严格)"(reference=w677, "ActiveCell"=w682, "CellBG"=w678) -> ()  [unwired: 1 in, 2 out]
        }
      }
    }
    n594 = property on="属性节点" class="MCListbox (严格)"(reference=w559, "ItemNames"="数据显示栏值") -> ()  [unwired: 1 in, 2 out]
    n595 = call "map.vi"("WebBrowser"="WebBrowser", "纬度"=w554, "经度"=w555) -> ()
    n596 = local read "状态"() -> (w576:string)
    n597 = local read "经度"() -> (w575:string)
    n598 = local read "纬度"() -> (w574:string)
    n599 = Match Pattern(string=w584, regular expression="$GPGGA,") -> (after substring=w588:string, offset past match=w586:i32)  [unwired: 1 in, 2 out]
    n600 = And(x=w551, y=w548) -> (x .and. y?=w550:bool)
    n601 = Bundle("状态"=w576, "经度"=w575, "纬度"=w574, "UTC时间"=w573) -> (→"GPS":T22)  [unwired: 1 in]
    n602 = Not Equal?(x=w586, y=-1) -> (x != y?=w587:bool)
    n603 = case shown="真" w550 {
      frame False {
      }
      frame True {
        n604 = Not(x="主摄像头开关") -> (.not. x?=w701:bool)
        n605 = call "Vision Acquisition"("Stop (F)"=w701) -> ("Image Out"=→"主摄像头":T8)  [unwired: 24 in, 2 out]
      }
    }
    n606 = case shown="真" w587 {
      tunnel: w588 -> [_ w945]
      frame False {
      }
      frame True {
        n607 = String Subset(string=w945, offset (0)=37, length (rest)=1 ("offset (0)")) -> (substring=w940:string)
        n608 = String Subset(string=w945, offset (0)=10, length (rest)=10 ("length (rest)")) -> (substring=w962:string)
        n609 = String Subset(string=w945, offset (0)=23, length (rest)=11 ("length (rest)")) -> (substring=w959:string)
        n610 = String Subset(string=w945, offset (0)=0, length (rest)=2 ("offset (0)")) -> (substring=w954:string)
        n611 = String Subset(string=w945, offset (0)=2, length (rest)=2 ("offset (0)")) -> (substring=w953:string)
        n612 = String Subset(string=w945, offset (0)=4, length (rest)=2 ("offset (0)")) -> (substring=w952:string)
        n613 = Concatenate Strings(w954, "时", w953, "分", w952, "秒") -> (→"UTC时间":string)
        n614 = Decimal String To Number(string=w940) -> (number=w939:i32)  [unwired: 2 in, 1 out]
        n615 = Fract/Exp String To Number(string=w962) -> (number=w966:dbl)  [unwired: 3 in, 1 out]
        n616 = Fract/Exp String To Number(string=w959) -> (number=w963:dbl)  [unwired: 3 in, 1 out]
        n617 = Multiply(x=w966, y=0.01) -> (x*y=w968:dbl)
        n618 = Multiply(x=w963, y=0.01) -> (x*y=w965:dbl)
        n619 = Index Array(array="GPS状态", index=w939) -> (element=→"状态":string)
        n620 = Number To Fractional String(number=w968) -> (F-format string=→"纬度":string)  [unwired: 3 in]
        n621 = Number To Fractional String(number=w965) -> (F-format string=→"经度":string)  [unwired: 3 in]
        "GPGGA" <- w945
      }
    }
    n622 = String Length(string=w569) -> (length=w568:i32)
    n623 = Greater Than 0?(x=w568) -> (x > 0?=w567:bool)
    n624 = property on="主摄像头" class="Bool (严格)"("Value"=w567) -> ()  [unwired: 2 in, 2 out]
  }
  n625 = VISA Close(VISA resource name=w14, error in (no error)=w13) -> (error out=w15:errorcluster)
  n626 = Unregister For Events(event registration refnum=w5, error in=w2) -> (error out=w3:errorcluster)
  n627 = call <vilib>:"Simple Error Handler.vi"("error in (no error)"=w15) -> ()  [unwired: 4 in, 5 out]
  n628 = Destroy User Event(user event=w1, error in=w3) -> ()  [unwired: 1 out]
  "报警历史" <- w6
  "报警数" <- w4
